vi "Real Time.vi"() -> ()   [LabVIEW 2022 SP3]
uses:
  ScanningControl/Motion Controllers/-MotionRoutines/MotionGlobals.vi
  <instrlib>/niScope/Controls/niScope input clock source.ctl
  ScanningControl/Pulsers/pulser.ctl
  ScanningControl/-ScanSystem/Controls/location.ctl
  ScanningControl/Motion Controllers/NI_controller/-NI_MotionRoutines/MotionSys.ctl
  <vilib>/Motion/FlexMotion/FunctionsVIs/Trajectory.llb/Load Acceleration/Deceleration.flx
  ScanningControl/-ScanSystem/Controls/ScanType2.ctl
  <vilib>/Utility/miscctls.llb/LVRectTypeDef.ctl
  <vilib>/ptbypt/NI_PtbyPt.lvlib
  <vilib>/picture/picture.llb/imagedata.ctl
  Annular Array/-AnnularRoutines/ArrayGeometry.ctl
  ScanningControl/Digitizers/-DigitizerRoutines/Digitizer.ctl
  <vilib>/Utility/miscctls.llb/LVBoundsTypeDef.ctl
  ScanningControl/Digitizers/-DigitizerRoutines/DigitizerGlobals.vi
  ScanningControl/Pulsers/PulserGlobals.vi
  Patient Routines/PatientGlobals.vi
  Annular Array/-AnnularRoutines/TransGeometry.ctl
  ScanningControl/Motion Controllers/Galil/Command Menu.ctl
  Annular Array/-AnnularRoutines/AnnularArray.ctl
panel:
  in  "Ann Array Params":T1={"Synth Foc?"=FALSE, "Focal Zones"=41, "Switch T/R"=0, "Trans Geometry (mm)"={"Transducer"=0, "Geo Focus"=12.0, "a (radius)"=3.0, "# of rings"=5, "kerf space "=0.1, "Center Freq"=12.0}, "Sub Ap Excite?"=FALSE, "Full Array Scan?"=FALSE, "Xmt/Rcv"={"XMIT"=[TRUE, TRUE, TRUE, TRUE, TRUE], "RCV"=[TRUE, TRUE, TRUE, TRUE, TRUE]}, "PulseSpacing (us)"=0.0, "Xmit Ring"=0, "XMIT CHS"=0, "RCV CHS"=0, "GPU?"=FALSE, "Save TIFF?"=FALSE, "downfactor"=1, "RCV 1CH"=0} {"RCV 1CH" items=["All", "1", "2", "3", "4", "5"]; "Trans Geometry (mm)"."Transducer" items=["6D 12R 40 MHz"=0, "10D 31R 20 MHz"=1, "10D 23R 20 MHz"=2, "6D 23R 40 MHz"=3, "4.5D 10.7R 40 MHz"=4, "9D 23.5R 20 MHz"=5, "9D 25.8R 20MHz"=6, "Enter"=99]; "Switch T/R" min=1 max=5 step=1}
  out "File Name":string="2015_000"
  in  "ExitSendCmd":bool
  in  "Sector":bool
  in  "Visible":bool
  in  "Center":bool
  in  "c (m/s)":dbl=1485.0
  out "append letter":i8=65
  in  "Scale (dB)":cluster{i32, i32}(slide)={-55, 0}
  out "Raw data":dbl[][](graph)
  in  "Tab Control":enum32{"Main Control", "Special Settings"}(tab)
  in  "Mode":T4(ring)
  in  "Save All Queue":bool
  out "fps":dbl format="%.1g"
  out "InQueue":i32
  in  "Patient Info":bool
  in  "Plane":i8(knob)=1 min=1 max=12 step=1 scale=0.0..12.0
  in  "View Queue":bool
  in  "Save All Real Time":bool
  in  "Save Raw":bool
  out "No data\nEntering\nQueue":bool
  in  "Pause":bool=TRUE
  in  "Flush Queue":bool
  in  "Image Scaling":T5(radio)
  in  "go":bool
  in  "Scan Location":enum32{"Radio Selection 1", "Radio Selection 2"}(radio)
  in  "Daxsonics Settings":T6={"Freq (MHz) "=20, "Amp (V)"=0, "Gain (dB)"=22} {"Freq (MHz)" items=["50"=50, "45"=45, "40"=40, "35"=35, "30"=30, "25"=25, "20"=20, "17"=17, "15"=15, "12"=12, "10"=10, "8"=8, "6"=6, "4"=4]; "Amp (V)" items=["100"=100, "95"=95, "90"=90, "85"=85, "80"=80, "75"=75, "70"=70, "65"=65, "60"=60, "55"=55, "50"=50, "45"=45, "40"=40, "35"=35, "30"=30, "25"=25, "20"=20, "15"=15, "10"=10, "0"=0]; "Gain (dB)" items=["45"=45, "42"=42, "39"=39, "36"=36, "33"=33, "30"=30, "27"=27, "24"=24, "21"=21, "18"=18, "15"=15, "12"=12, "9"=9, "6"=6, "3"=3, "0"=0]}
  out "Process backlog":i32
  in  "Accel":dbl(slide)=100.0 scale=1000000.0..7000000.0 scale format="%#_6e"
  in  "Adjust fps (%)":i16(slide)=100 min=0 max=150 step=5 scale=0.0..150.0
  in  "Xtra delay (us)":dbl=10.0
  in  "LowTime":dbl=0.01
  in  "Gate Length":dbl=0.19 format="%.6f"
  in  "Filter?":bool=TRUE
  in  "Dig Scale":dbl(ring)=0.4 items=["10 V"=10.0, "4 V"=4.0, "2 V"=2.0, "1 V"=1.0, "400 mV"=0.4, "200 mV"=0.2, "100 mV"=0.1]
  in  "RF data Sampling":T7={"Sampling Rate"=100.0, "Ref Delay (ms)"=0.0, "rf points per line"=2048} {"rf points per line" min=1; "Ref Delay (ms)" format="%.2f"}
  out "Frame":i32
  out "Sat Ct":u16(slide) scale=0.0..400.0
  in  "N":u8=100 min=1 max=100 step=1
  in  "Xmt/Rcv":cluster{"XMIT":bool[], "RCV":bool[]}={"XMIT"=[TRUE, TRUE, TRUE, TRUE, TRUE], "RCV"=[TRUE, TRUE, TRUE, TRUE, TRUE]}
  in  "Focal Zones":i16
  in  "GPU?":bool
  # "Ruler"
  # "© 2011-2015 Riverside Research Institute"
  # "Daxsonics"
  # "View"
  # "Data Archiving"
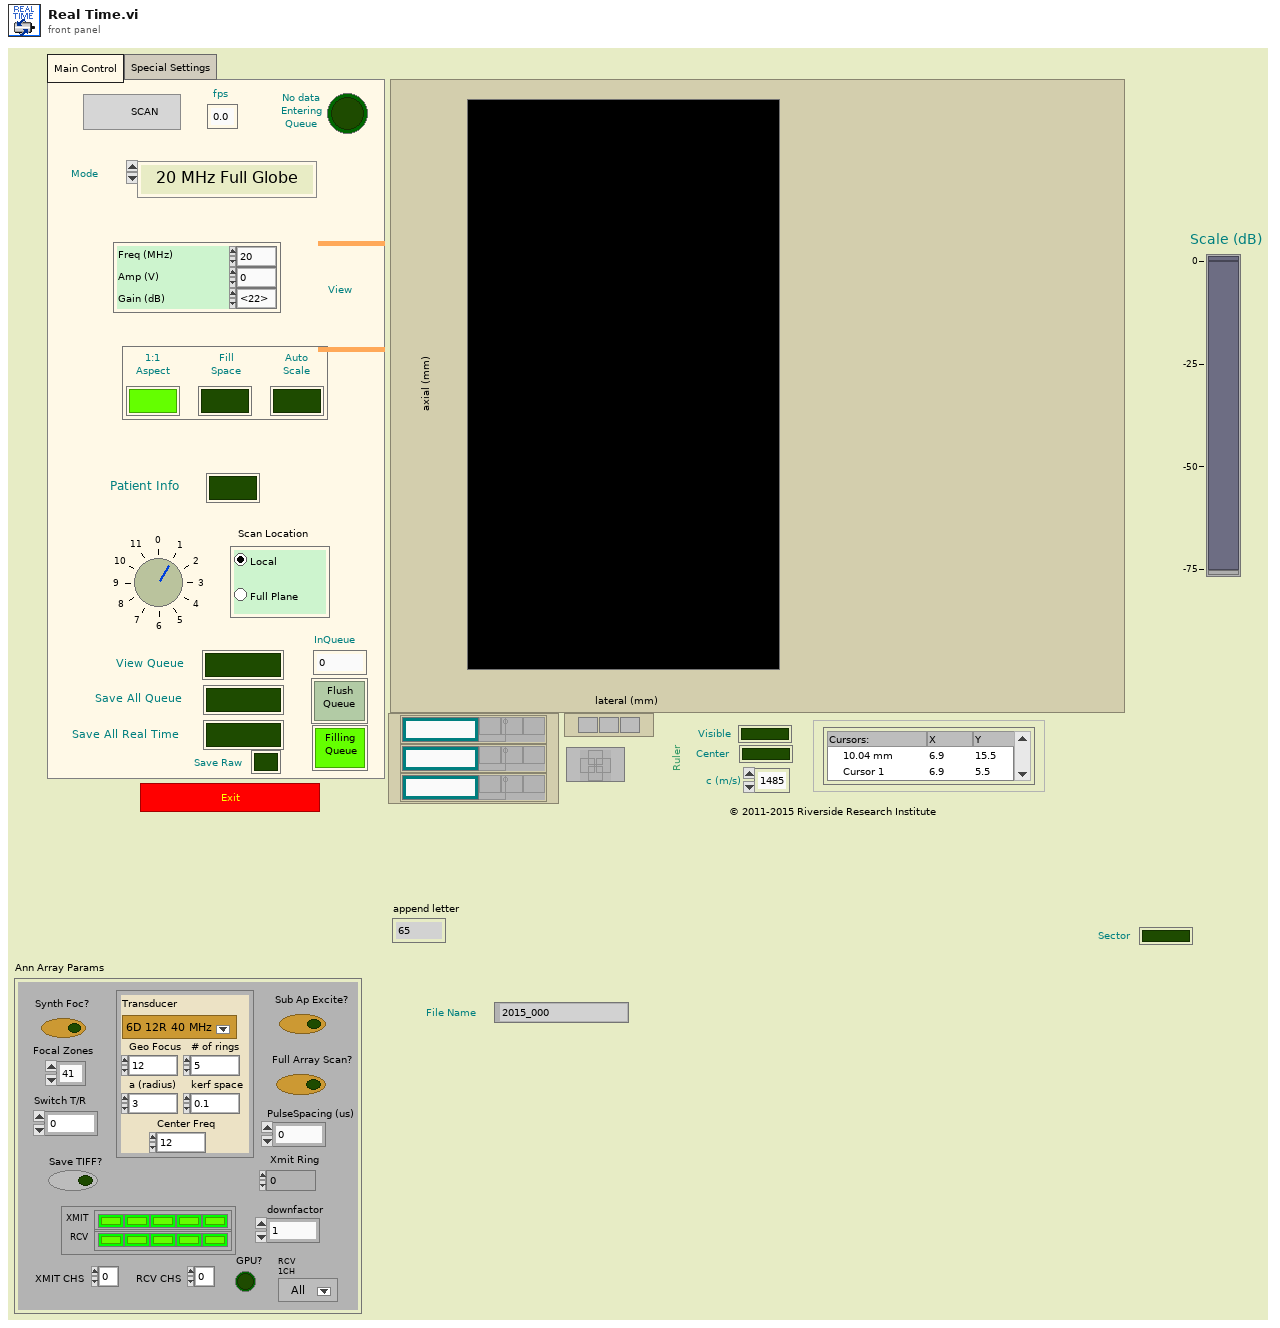
[diagram p1: front panel]
types:
  T1 = typedef "AnnularArray.ctl" = cluster{"Synth Foc?":bool, "Focal Zones":i16, "Switch T/R":i16, "Trans Geometry (mm)":T2, "Sub Ap Excite?":bool, "Full Array Scan?":bool, "Xmt/Rcv":cluster{"XMIT":bool[], "RCV":bool[]}, "PulseSpacing (us)":sgl, "Xmit Ring":i32, "XMIT CHS":u8, "RCV CHS":u8, "GPU?":bool, "Save TIFF?":bool, "downfactor":i32, "RCV 1CH":u16}
  T2 = typedef "TransGeometry.ctl" = cluster{"Transducer":T3, "Geo Focus":dbl, "a (radius)":dbl, "# of rings":i32, "kerf space ":dbl, "Center Freq":dbl}
  T3 = typedef "ArrayGeometry.ctl" = u16
  T4 = enum16{"20 MHz Full Globe", "20 MHz Anterior", "20 MHz Posterior", "New 20 MHz Full Globe", "New 20 MHz Anterior", "New 20 MHz Posterior", "F2 40 MHz", "F2 40 MHz Deep", "F3 20 MHz", "F3 20 MHz Deep", "Aviso Probe"}
  T5 = enum32{"1:1\nAspect", "Fill\nSpace", "Auto\nScale"}
  T6 = cluster{"Freq (MHz) ":u16, "Amp (V)":u16, "Gain (dB)":u16}
  T7 = cluster{"Sampling Rate":dbl, "Ref Delay (ms)":dbl, "rf points per line":i32}
  T8 = typedef "Digitizer.ctl" = enum16{"Acqiris Digitizer", "NI Digitizer", "LeCroy", "GaGe", "AlazarTech", "No Digitizer", "Teledyne"}
  T9 = typedef "LVBoundsTypeDef.ctl" = cluster{"Width":u32, "Height":u32}
  T10 = typedef "LVRectTypeDef.ctl" = cluster{"Left":i16, "Top":i16, "Right":i16, "Bottom":i16}
  T11 = typedef "pulser.ctl" = enum16{"Pan 5900", "Daxsonics", "Agilent 33xxx", "UTEX", "JSR", "WMC Mono-Cycle", "No Pulser", "NYU AVTECH", "Tabor W1281A", "Pan 5800", "Unlisted", "Tabor WX2182B"}
  T12 = typedef "MotionSys.ctl" = enum16{"MM3000", "NI 735x", "Newport ESP", "No Motion Card", "Galil"}
  T13 = typedef "location.ctl" = enum16{"Automatic", "WCM Main", "Hawaii", "Columbia MM3000", "Columbia  NI System", "NYU", "RRI 2", "UHI Allen", "CUMC RT", "Chiba", "Stony Brook", "WCM Microscopy", "WCM Aeoretch", "WCM Optics Lab", "WCM Main 2Axis", "WCM Rotation", "WCM SAM SMAC", "SERI GP"}
  T14 = typedef "DigitizerSettings.ctl" = cluster{"Digitizer delay (us) ":dbl, "rf points per line":i32, "lines per plane":i32, "Samp Rate (Hz)":dbl, "Additional dig delay (us)":dbl, "Voltage Scale":dbl, "Pre-Looks":i32, "Offset delay (us)":dbl, "bits A/D":i8, "Avg Num":i32, "DigTimeOut":sgl, "Rel Dig Delay":sgl, "Dig Ch":i32, "LeCroyCluster":cluster{"LeCroy Channels":bool[], "LC read pt offset":dbl, "Sweep Avg":bool}, "Main Digitizer":T8, "Dig Config":T15, "Digitizer ID Cluster":T16, "Trigger Settings":cluster{"Trig Source":u16, "Trig Coupling":u16, "Trig Slope":u16, "Level (mV)":dbl}, "Bulk Acq":bool, "Bulk Start Indexes":i32[], "Data Ref RF":refnum<data-value>, "NI ID/Channel":cluster{"NI ID":refnum<k15>, "NI CH":i32}[], "Total Dig CH":i32, "Xtra Ann Trig delay (us)":dbl, "Fix Z Delay?":bool, "One Way Transmission?":bool, "Data Ref Log":refnum<data-value>}
  T15 = typedef "DigConfig.ctl" = enum16{"Single channel", "2 Chans w/ 2 Acqiris", "2 Chans w/ 1 Acqiris", "5-CH Pulser New", "5-CH pulser w/ ann array", "5-pass style ann array", "Empty"}
  T16 = typedef "DigitizerID.ctl" = cluster{"Acqiris/Alazar/SP ID":u32[], "NI Instr Handles":refnum<k15>[], "LeCroy VISA":refnum<visa-resource-name>, "GaGe Handle":cluster{"Handle":u32, "Sample size":u32, "Resolution":i32, "Offset":i32, "Channels":u32, "Boards":u32}, "ATS Ref":string, "Acqiris Address":string[], "ADQRef":refnum<k24>, "adq_cu_ptr":refnum<k24>}
  T17 = cluster{"DataBufferQ":refnum<queue>, "LastNQ":refnum<queue>, "LastNBMPQ":refnum<queue>, "SaveRawN":refnum<notifier>, "StopN":refnum<notifier>}
  T18 = typedef "imagedata.ctl" = cluster{"image type":i32, "image depth":i32, "image":u8[], "mask":u8[], "colors":u32[], "Rectangle":cluster{"left":i16, "top":i16, "right":i16, "bottom":i16}}
  T19 = cluster{"gain":dbl, bool, "wfm":i16[][], "Sat Pts":i32, bool}
  T20 = cluster{"Source":u16, "Coupling":u16, "Slope":u16, "Level":dbl}
  T21 = typedef "ScanType2.ctl" = enum16{"Therapy With Scan", "M scan", "M Scan With Therapy Burst", "1-D B Scan", "1-D B Scan With Therapy Burst", "2-D B Scan", "2-D B Scan With Therapy Burst", "Rotational Scan", "1-D B-Scan PRF", "2-D B-Scan PRF", "Real-Time Scan", "Contrast Agents", "1-D w/ Real-Time Set Up", "Dual Transducer", "Acoustic Microscopy", "Hydrophone Scanning"}
  T22 = enum16{"Home", "Index", "Center", "Forward Limit", "Reverse Limit", "Run Sequence"}
  T23 = typedef "Command Menu.ctl" = enum16{"CommandPassThrough", "Abort Motion", "Define Pos", "Velocity", "Acceleration", "Deceleration", "Position Rel", "Postion Abs", "Begin Move", "KI", "KD", "KP", "IL", "Config I/O", "Set Bit", "Clear Bit", "Motor Off", "Moto On", "Status", "Execute", "Halt Execute", "HX Status", "Tell Velocity", "Check Motion", "BreakPoint", "Tell Position", "Current Code Line", "Tell Switches", "OC Force On", "OC Off"}
  T24 = cluster{"low cutoff":i32, "order":i32, "high cutoff":i32}
  T25 = cluster{"Source":u16, "Coupling":u16, "Slope":u16, "Level (mV)":dbl}
  T26 = cluster{"Voltage Scale":dbl, "Offset":dbl, "Coupling":u16}
  T27 = typedef "niScope input clock source.ctl" = u16
  T28 = typedef "LVStringsAndValuesArrayTypeDef_DBL.ctl" = cluster{"String":string, "Value":dbl}[]
  T29 = typedef "LVStringsAndValuesArrayTypeDef_U16.ctl" = cluster{"String":string, "Value":u16}[]
  T30 = typedef "Dax_Control_Cluster.ctl" = cluster{"Freq (MHz) ":u16, "Voltage (V)":u16, "Gain (dB)":u16}
  T31 = typedef "MotionParameters.ctl" = cluster{"No Motion?":bool, "Motion System":T12, "Motion Bd ID":u8, "Motion Profile":string, "# Axis":i8, "Reverse Z axis?":bool, "SMAC Axis":u16, "scan pair":T32, "RT fps":sgl, "Steps per mm":i32[], "Motor Parameters":cluster{"velocity ct/s":dbl[], "accel ct/s^2":dbl[]}, "One Way Scan":bool, "Reverse One Way Scan":bool, "Global Position (mm)":dbl[], "Plane":i32, "Distance between\nscan lines (um)":sgl, "Distance between\nscan planes (um)":sgl, "number of scan planes":i32, "Total steps in line":i32, "Xtra plane\ndistance  (um)":i32, "Xtra planes ":i32, "Add Axis":bool, "overshoot cts":i32, "BKPT Shift":i32, "Scan Start Time (ms)":u32, "ESP VISA":refnum<visa-resource-name>, "3rd Axis":T33, "GL Ref Out":refnum<k7>, "Galil Address":string}
  T32 = typedef "ScanAxis.ctl" = enum16{"y-(x) scan", "x-(y) scan", "z-(x) scan", "z-(y) scan", "y-(z) scan", "x-(z) scan", "w-(x) scan", "w-(y) scan", "w-(z) scan", "x-(w) scan", "y-(w) scan", "z-(w) scan"}
  T33 = typedef "3rdAxis.ctl" = u16
  T34 = typedef "Bd Id Out" = u8
  T35 = typedef "Resource Out (Enum).flx" = u16
  T36 = typedef "AxisOrVectorSpaceControl To Control.flx" = u16
  T37 = typedef "GL Axis Control.ctl" = u16
  T38 = cluster{"FIR Windowed Coefficients":dbl[], "Filter Prams":cluster{"low cutoff":i32, "order":i32, "high cutoff":i32}}
  T39 = cluster{"gain":dbl, bool, "wfm":i16[][], "max queue size (-1, unlimited)":i32, bool}
  T40 = cluster{"Y Scale Offset":dbl, "Y Scale Multi":dbl, "X Scale Offset":dbl, "X Scale Multi":dbl, "Gate Distance":dbl}
  T41 = typedef "PatientInfoDef.ctl" = cluster{"Eye Selector":enum32{"Left", "Right"}, "Plane":i8, "First Name":string, "Last Name":string, "Notes":string, "Patient ID":string, "Scan Location":enum32{"Radio Selection 1", "Radio Selection 2"}}
  T42 = typedef "LVPointDoubleTypeDef.ctl" = cluster{"Cursor X":dbl, "Cursor Y":dbl}
  T43 = typedef "LVRangeTypeDef.ctl" = cluster{"Minimum":dbl, "Maximum":dbl, "Increment":dbl, "Minor Increment":dbl, "Start":dbl}
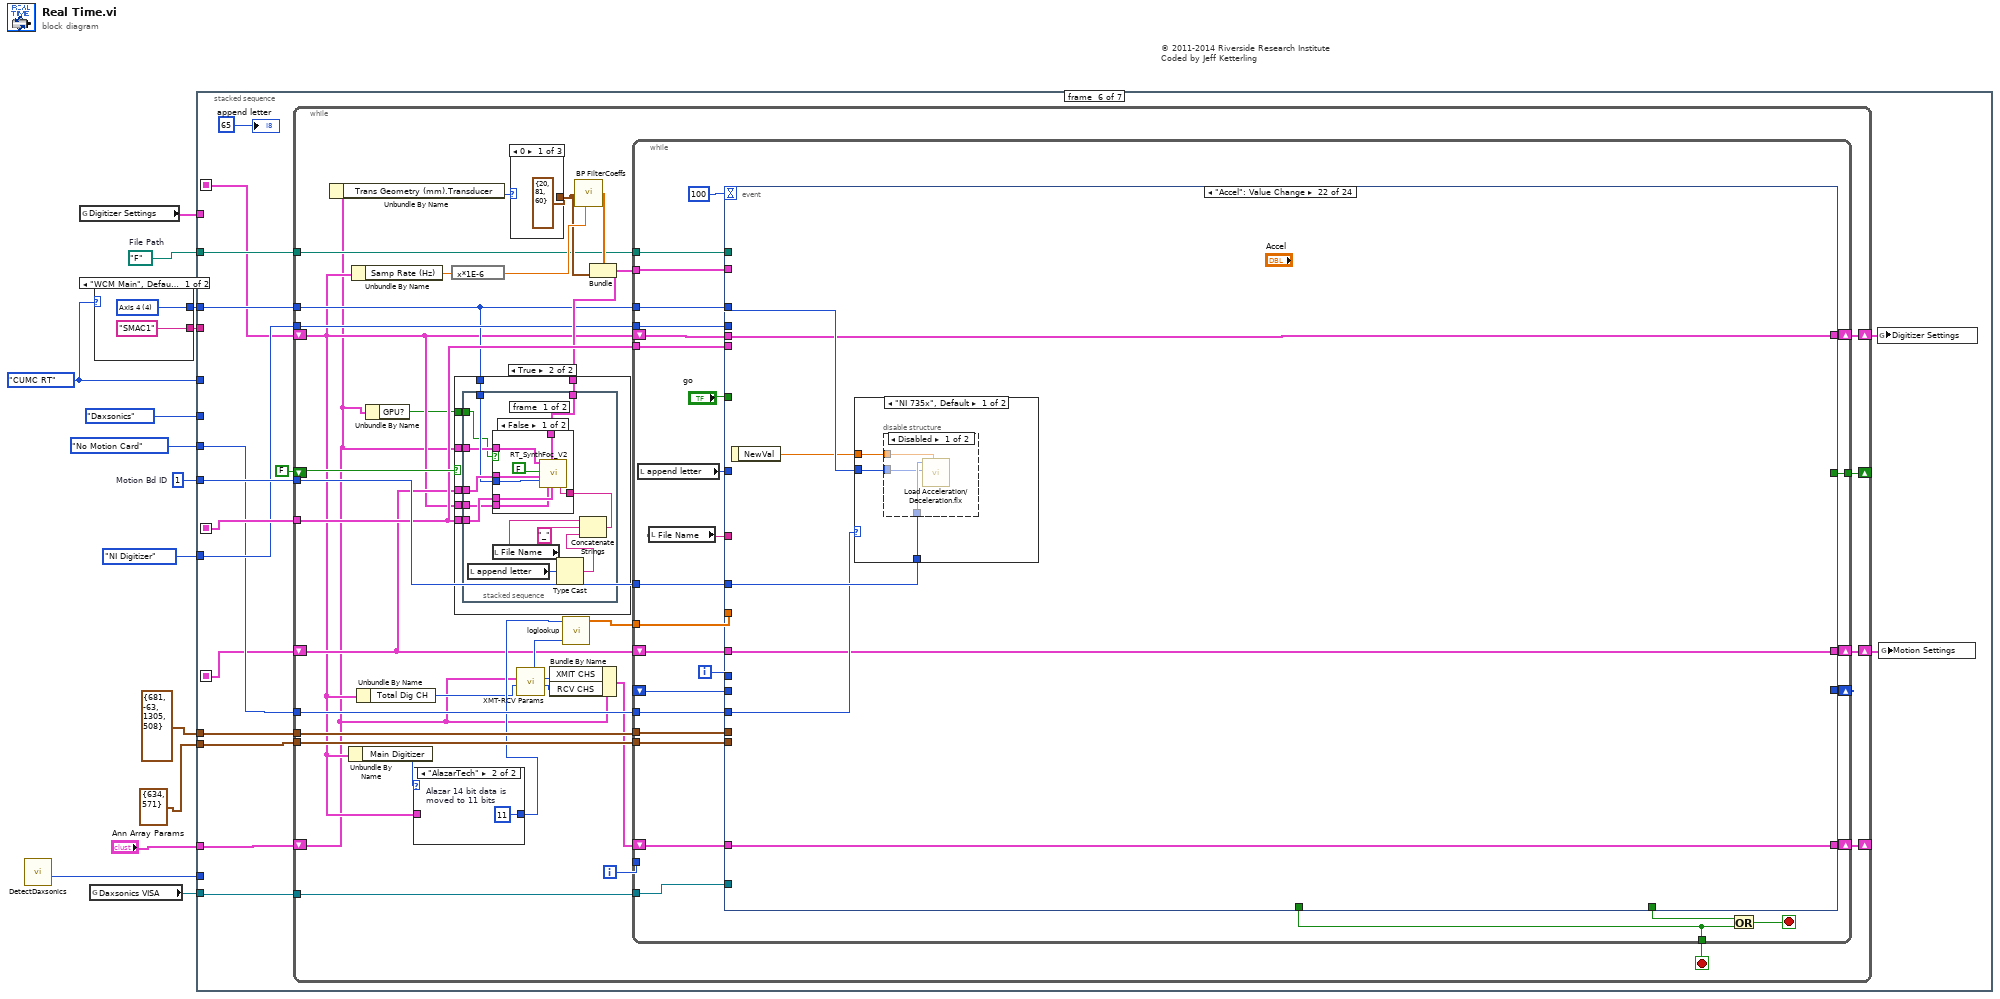
[diagram p0: block diagram]
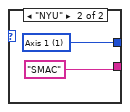
[diagram p2: hidden frame]
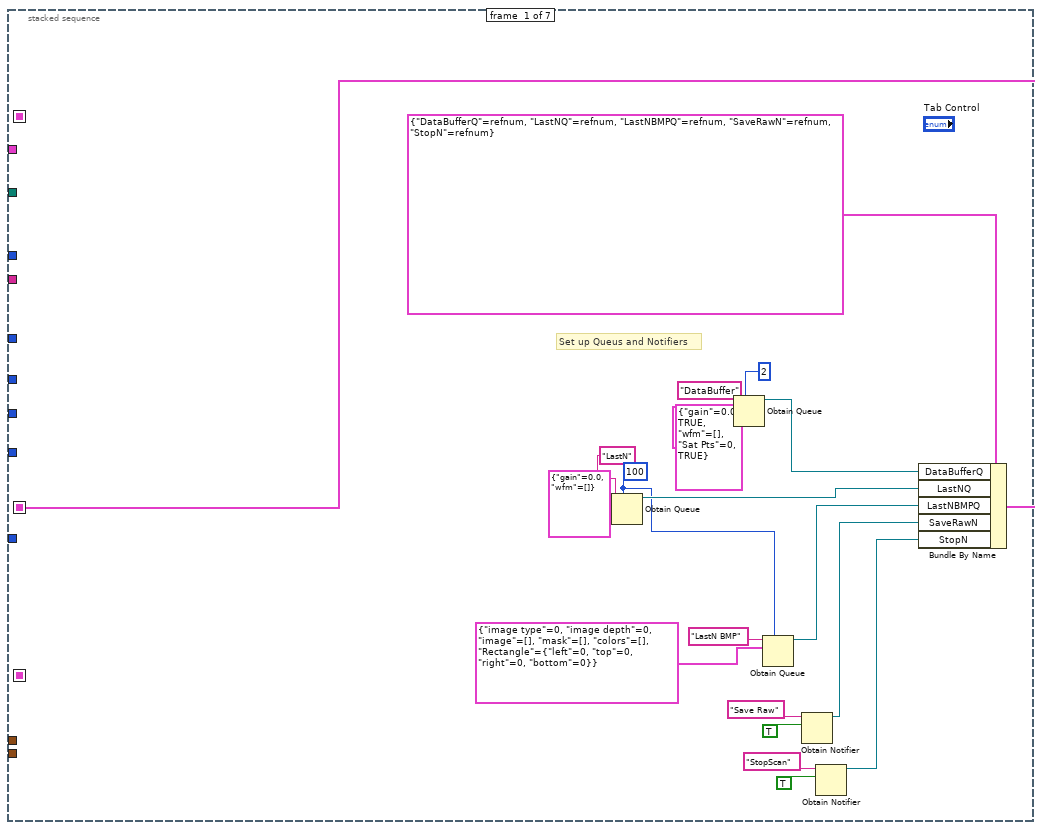
[diagram p3: hidden frame]
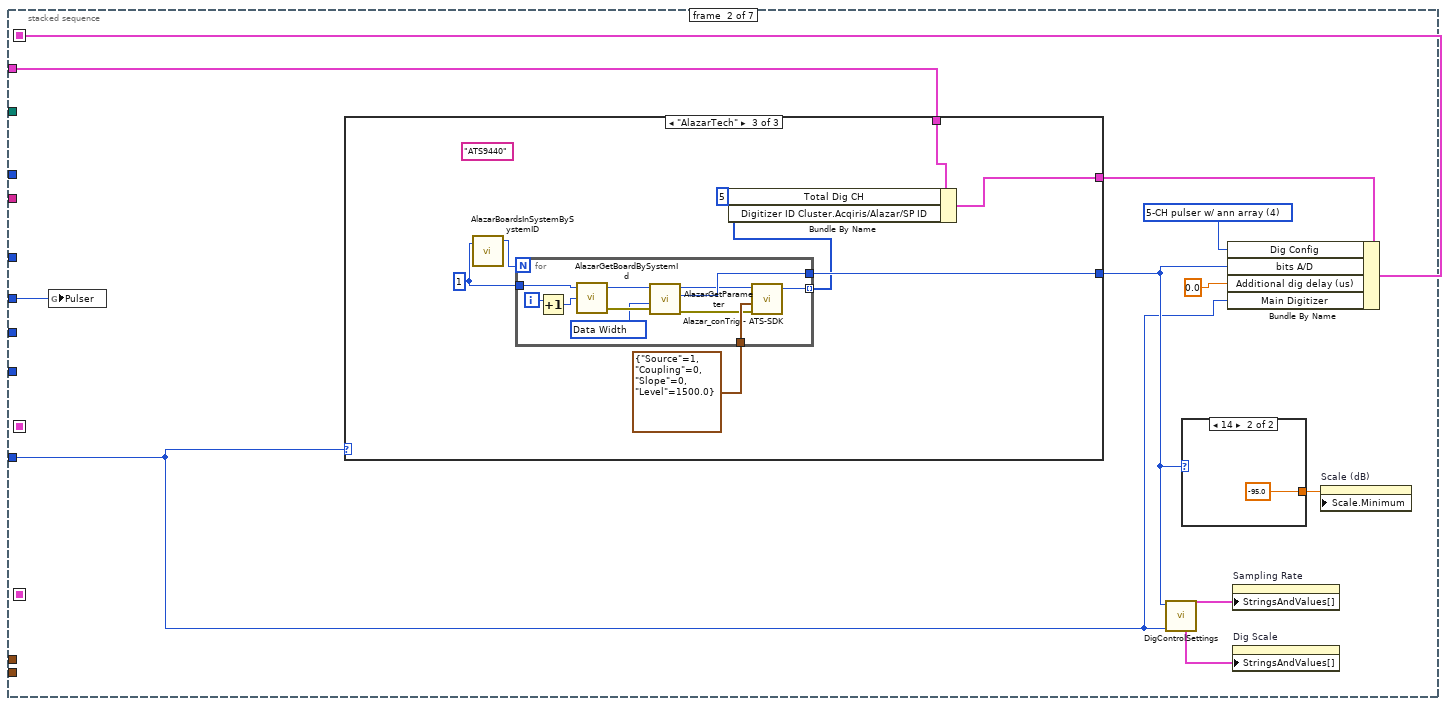
[diagram p4: hidden frame]
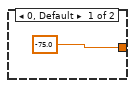
[diagram p5: hidden frame]
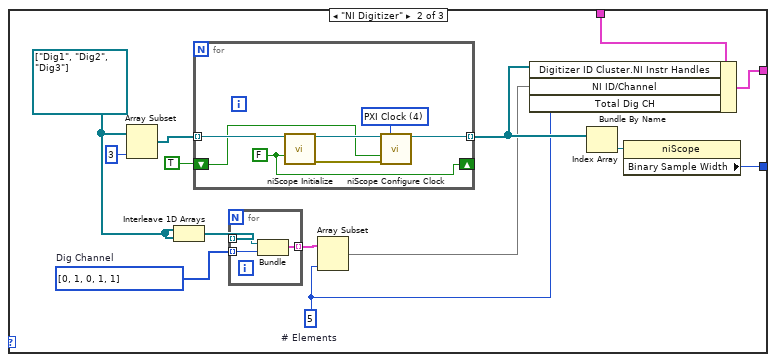
[diagram p7: hidden frame]
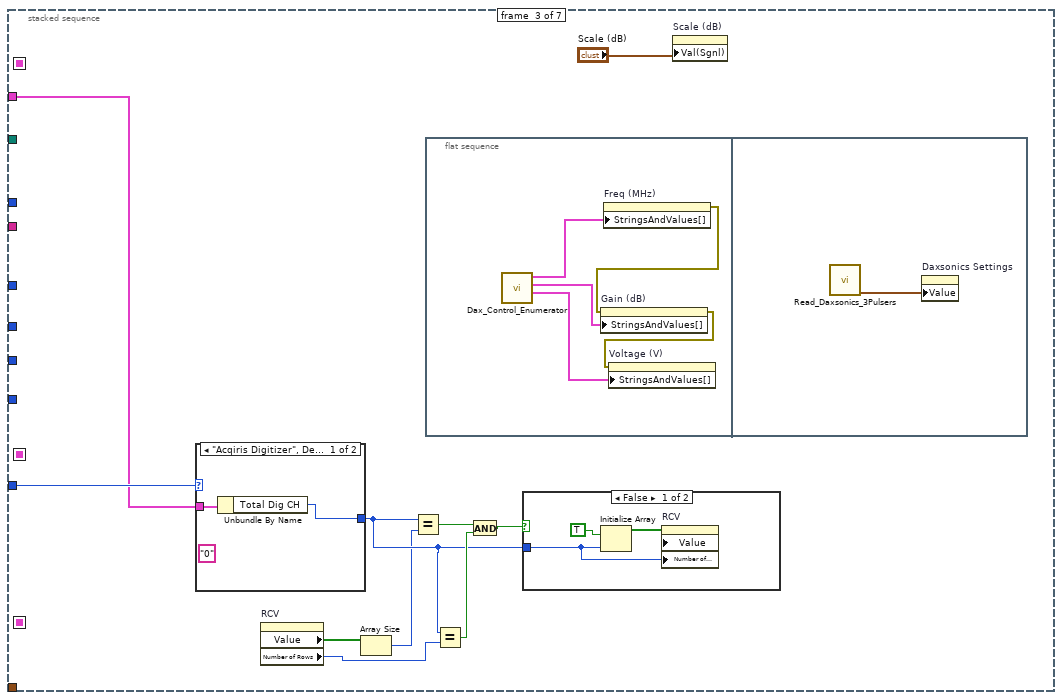
[diagram p8: hidden frame]
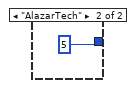
[diagram p10: hidden frame]
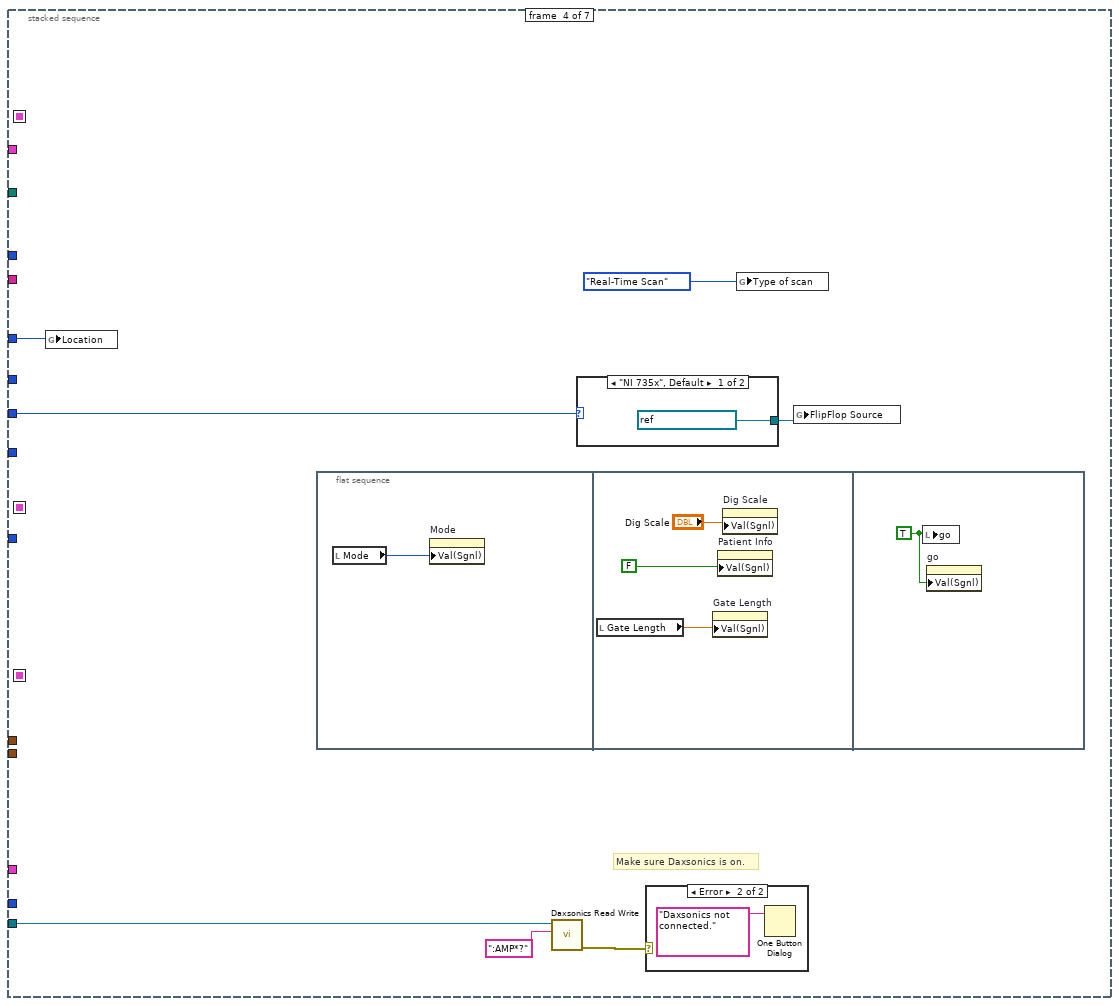
[diagram p11: hidden frame]
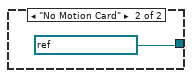
[diagram p12: hidden frame]
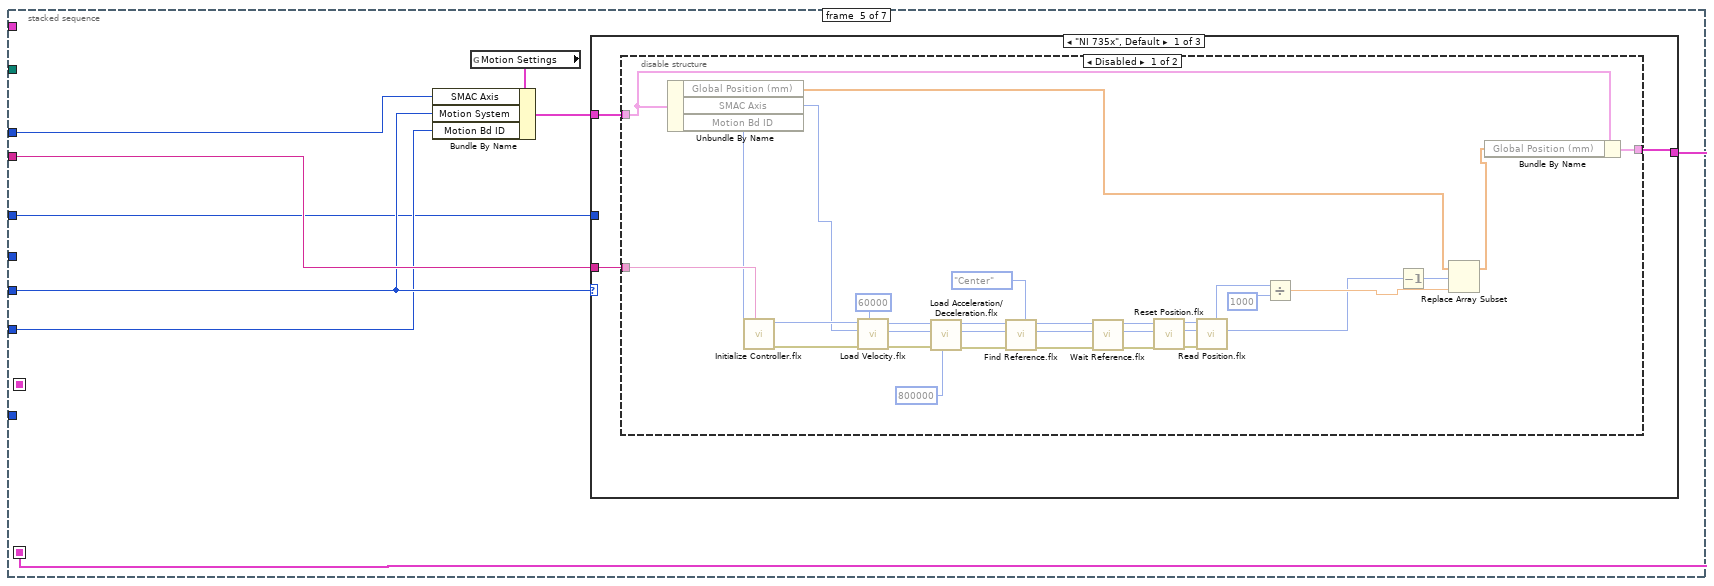
[diagram p14: hidden frame]
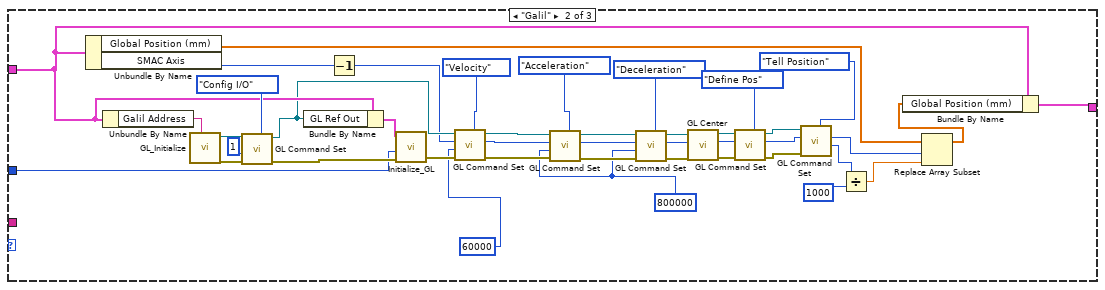
[diagram p16: hidden frame]
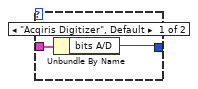
[diagram p18: hidden frame]
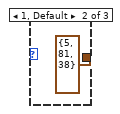
[diagram p19: hidden frame]
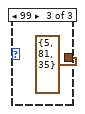
[diagram p20: hidden frame]
diagram:
  w8 = path "F:/"  # File Path
  w12 = location."CUMC RT" ("Location")
  w14 = u8 1  # Motion Bd ID
  # "© 2011-2014 Riverside Research Institute\nCoded by Jeff Ketterling"
  n1 = call "DetectDaxsonics.vi"() -> ("Trig Slope"=w2:u16)  [unwired: 10 in, 1 out]
  n2 = global read "DigitizerGlobals.vi" "Digitizer Settings"() -> (w7:T14)
  n3 = global read "PulserGlobals.vi" "Daxsonics VISA"() -> (w1:refnum<visa-resource-name>)
  n4 = case shown="\"WCM Main\", Default" w12 {
    tunnel: [w16 w18] -> w13
    tunnel: ["SMAC1" "SMAC"] -> w10
    frame "WCM Main", Default {
      w16 = u16 4 items=["Axis 1"=1, "Axis 2"=2, "Axis 3"=3, "Axis 4"=4, "Axis 5"=5, "Axis 6"=6, "Axis 7"=7, "Axis 8"=8, "Vector Space 1"=17, "Vector Space 2"=18, "Vector Space 3"=19, "Vector Space 4"=20] ("Axis")
    }
    frame "NYU" {
      w18 = u16 1 items=["Axis 1"=1, "Axis 2"=2, "Axis 3"=3, "Axis 4"=4, "Axis 5"=5, "Axis 6"=6, "Axis 7"=7, "Axis 8"=8, "Vector Space 1"=17, "Vector Space 2"=18, "Vector Space 3"=19, "Vector Space 4"=20] ("Axis")
    }
  }
  n5 = stacked-sequence {
    seq-local: [w24 _ _ _ _ _ _] -> [_ _ _ _ _ w226 w977]
    seq-local: [_ w44 _ _ _ _ _] -> [_ _ _ _ _ w222 w974]
    seq-local: [_ _ _ _ w133 _ _] -> [_ _ _ _ _ w221 _]
    tunnel: w14 -> [_ _ _ _ w135 w232 _]
    tunnel: MotionSys."No Motion Card" ("Motion System") -> [_ _ _ w117 w136 w224 _]
    tunnel: w12 -> [_ _ _ w121 w131 _ _]
    tunnel: T9 {"Width"=634, "Height"=571} ("Plot Area:Size") -> [_ _ _ _ _ w230 w985]
    tunnel: T10 {"Left"=681, "Top"=-63, "Right"=1305, "Bottom"=508} ("Plot Area Bounds") -> [_ _ _ _ _ w229 w986]
    tunnel: w13 -> [_ _ _ _ w137 w228 _]
    tunnel: Digitizer."NI Digitizer" ("Main Digitizer") -> [_ w40 w102 _ _ w225 w976]
    tunnel: w10 -> [_ _ _ _ w138 _ _]
    tunnel: w8 -> [_ _ _ _ _ w223 _]
    tunnel: w7 -> [_ w43 w94 _ _ _ _]
    tunnel: pulser."Daxsonics" ("Pulser") -> [_ w38 _ _ _ _ _]
    tunnel: "Ann Array Params" -> [_ _ _ _ _ w218 _]
    tunnel: w2 -> [_ _ _ _ _ _ _]
    tunnel: w1 -> [_ _ _ w116 _ w217 _]
    frame #0 {
      w19 = 100 ("max queue size (-1, unlimited)")
      # "Set up Queus and Notifiers"
      n6 = Obtain Queue ("LastN")(max queue size (-1, unlimited)=w19, name (unnamed)="LastN", element data type=cluster{"gain":dbl, "wfm":i16[][]} {"gain"=0.0, "wfm"=[]}) -> (queue out=w25:refnum<queue>)  [unwired: 2 in, 2 out]
      n7 = Obtain Queue(max queue size (-1, unlimited)=2, name (unnamed)="DataBuffer", element data type=T19 {"gain"=0.0, TRUE, "wfm"=[], "Sat Pts"=0, TRUE}) -> (queue out=w20:refnum<queue>)  [unwired: 2 in, 2 out]
      n8 = Obtain Queue ("LastNBMP")(max queue size (-1, unlimited)=w19, name (unnamed)="LastN BMP", element data type=T18 {"image type"=0, "image depth"=0, "image"=[], "mask"=[], "colors"=[], "Rectangle"={"left"=0, "top"=0, "right"=0, "bottom"=0}} ("Image Data")) -> (queue out=w23:refnum<queue>)  [unwired: 2 in, 2 out]
      n9 = Obtain Notifier ("Raw eye")(name (unnamed)="Save Raw", notification data type=TRUE) -> (notifier out=w26:refnum<notifier>)  [unwired: 2 in, 2 out]
      n10 = Obtain Notifier ("Stop Scan")(name (unnamed)="StopScan", notification data type=TRUE) -> (notifier out=w22:refnum<notifier>)  [unwired: 2 in, 2 out]
      n11 = Bundle By Name(cluster=T17 {"DataBufferQ"=refnum, "LastNQ"=refnum, "LastNBMPQ"=refnum, "SaveRawN"=refnum, "StopN"=refnum} ("Qs and Notis"), "DataBufferQ"=w20, "LastNQ"=w25, "LastNBMPQ"=w23, "SaveRawN"=w26, "StopN"=w22) -> (w24:T17)
    }
    frame #1 {
      w39 = 4 items=["Single channel"=0, "2 Chans w/ 2 Acqiris"=1, "2 Chans w/ 1 Acqiris"=2, "5-CH pulser w/ ann array"=4, "5-pass style ann array"=5] ("Dig Config")
      n12 = global write "PulserGlobals.vi" "Pulser"(w38) -> ()
      n13 = case shown="\"AlazarTech\"" w40 {
        tunnel: [_ w61 w79] -> w45
        tunnel: w43 -> [_ w58 w82]
        tunnel: [_ w59 w81] -> w42
        frame "Acqiris Digitizer", Default {
        }
        frame "NI Digitizer" {
          w51 = 5  # # Elements
          w57 = i32[] [0, 1, 0, 1, 1]  # Dig Channel
          w53 = refnum<k15>[] ["Dig1", "Dig2", "Dig3"]
          n14 = Array Subset(array=w53, length=3) -> (w63:refnum<k15>[])  [unwired: 1 in]
          n15 = Interleave 1D Arrays(w53, w53) -> (w55:refnum<k15>[])
          n16 = for {
            tunnel: [w71] -> w60 mode=indexing
            tunnel: w63 -> [w70] mode=indexing
            shift-right: [w68] -> _
            shift-left: TRUE ("master enabled") -> [w69]
            w68 = FALSE ("reset device")
            w74 = T27 4 items=["None"=0, "RTSI Clock"=1, "PFI 0"=6, "PFI 1"=2, "PFI 2"=3, "PXI Clock"=4, "External"=5, "Clock In"=7] ("input clock source")
            n17 = call <instrlib>:"niScope Initialize.vi"("resource name"=w70, "reset device"=w68) -> ("instrument handle"=w72:refnum<k15>, "error out"=w73:errorcluster)  [unwired: 2 in, 10 out]
            n18 = call <instrlib>:"niScope Configure Clock.vi"("instrument handle"=w72, "input clock source"=w74, "master enabled"=w69, "error in"=w73) -> ("instrument handle out"=w71:refnum<k15>)  [unwired: 2 in, 9 out]
          }
          n19 = for {
            tunnel: w55 -> [w67] mode=indexing
            tunnel: w57 -> [w66] mode=indexing
            tunnel: [w65] -> w56 mode=indexing
            n20 = Bundle("resource name"=w67, w66) -> (w65:cluster{"resource name":refnum<k15>, i32})  [unwired: 1 in]
          }
          n21 = Array Subset(array=w56, length=w51) -> (w52:cluster{"resource name":refnum<k15>, i32}[])  [unwired: 1 in]
          n22 = Bundle By Name(cluster=w58, "Digitizer ID Cluster.NI Instr Handles"=w60, "NI ID/Channel"=w52, "Total Dig CH"=w51) -> (w59:T14)
          n23 = Index Array(array=w60) -> (element=w64:refnum<k15>)  [unwired: 1 in]
          n24 = property class="niScope"(reference=w64) -> ("Binary Sample Width"=w61:i32)  [unwired: 1 in, 2 out]
        }
        frame "AlazarTech" {
          w76 = u32 1 ("System ID")
          (unwired) "ATS9440" ("BoardToVerify")
          n25 = call "AlazarBoardsInSystemBySystemID.vi"("System ID"=w76) -> ("Board Count"=w77:u32)  [unwired: 1 in, 2 out]
          n26 = for {
            N: w77 -> [_]
            tunnel: [w90] -> w79
            tunnel: T20 {"Source"=1, "Coupling"=0, "Slope"=0, "Level"=1500.0} ("Trigger") -> [w88]
            tunnel: w76 -> [w84]
            tunnel: [w83] -> w75 mode=indexing
            i -> [w86]
            w91 = u32 268435465 items=["Data Width"=268435465, "Set/Get Async BuffSize"=268435513, "Set/Get Async Buffcount"=268435520, "Get Data Format"=268435522, "Get Samples Per Timestamp Clock"=268435524, "Get Records Captured"=268435525, "Get Async Buffers Pending"=268435536, "Get Async Buffers Pending Full"=268435537, "Get Async Buffers Pending Empty"=268435538, "ECC Mode"=268435528, "Get Aux Input Level"=268435529, "Get Channels Per Board"=268435568, "Pack Mode"=268435570, "Get FPGA Temperature"=268435584] ("Parameter")
            n27 = Increment(x=w86) -> (x+1=w85:i32)
            n28 = call "AlazarGetBoardBySystemId.vi"("Board ID"=w85, "System ID"=w84) -> ("error out"=w92:errorcluster, "Handle"=w93:u64)  [unwired: 1 in, 1 out]
            n29 = call "AlazarGetParameter.vi"("error in (no error)"=w92, "Parameter"=w91, "Handle"=w93) -> ("error out"=w87:errorcluster, "Value"=w90:i32, "Handle"=w89:u64)  [unwired: 1 in, 1 out]
            n30 = call "Alazar_conTrig - ATS-SDK.vi"("error in (no error)"=w87, "Trigger"=w88, "Handle in"=w89) -> ("Handle_Out"=w83:u32)  [unwired: 2 in, 1 out]
          }
          n31 = Bundle By Name(cluster=w82, "Total Dig CH"=5, "Digitizer ID Cluster.Acqiris/Alazar/SP ID"=w75) -> (w81:T14)
        }
      }
      n32 = call "DigControlSettings.vi"(8:w40, 11:w45) -> ("Sampling Rates"=w47:T28, "Voltage Scale"=w48:T28)  [unwired: 5 in, 3 out]
      n33 = case shown="14" w45 {
        tunnel: [-75.0 ("Scale.Range:Maximum") -95.0 ("Scale.Range:Maximum")] -> w46
        frame 0, Default {
        }
        frame 14 {
        }
      }
      n34 = Bundle By Name(cluster=w42, "Dig Config"=w39, "bits A/D"=w45, "Additional dig delay (us)"=0.0 ("Additional dig delay (ms)"), "Main Digitizer"=w40) -> (w44:T14)
      n35 = property on="Sampling Rate" class="Ring (strict)"("StringsAndValues[]"=w47) -> ()  [unwired: 2 in, 2 out]
      n36 = property on="Dig Scale" class="Ring (strict)"("StringsAndValues[]"=w48) -> ()  [unwired: 2 in, 2 out]
      n37 = property on="Scale (dB)" class="Slide (strict)"("Scale.Minimum"=w46) -> ()  [unwired: 2 in, 2 out]
    }
    frame #2 {
      n38 = case shown="\"Acqiris Digitizer\", Default" w102 {
        tunnel: [w107 5] -> w98
        tunnel: w94 -> [w108 _]
        frame "Acqiris Digitizer", Default {
          (unwired) "0" ("Active Channel")
          n39 = Unbundle By Name(w108) -> ("Total Dig CH"=w107:i32)
        }
        frame "AlazarTech" {
        }
      }
      n40 = property on="RCV" class="Arr (strict)"() -> ("Value"=w103:bool[], "Number of Rows"=w96:u32)  [unwired: 2 in, 2 out]
      n41 = Array Size(array=w103) -> (size(s)=w97:i32)
      n42 = Equal?(x=w98, y=w97) -> (x = y?=w100:bool)
      n43 = flat-sequence {
        frame #0 {
          n44 = call "Dax_Control_Enumerator.vi"() -> ("Voltage"=w114:T29, "Gain"=w113:T29, "Freq"=w112:T29)  [unwired: 9 in]
          n45 = property on="Freq (MHz)" class="Ring (strict)"("StringsAndValues[]"=w112) -> (error out=w111:errorcluster)  [unwired: 2 in, 1 out]
          n46 = property on="Gain (dB)" class="Ring (strict)"(error in=w111, "StringsAndValues[]"=w113) -> (error out=w110:errorcluster)  [unwired: 1 in, 1 out]
          n47 = property on="Voltage (V)" class="Ring (strict)"(error in=w110, "StringsAndValues[]"=w114) -> ()  [unwired: 1 in, 2 out]
        }
        frame #1 {
          n48 = call "Read_Daxsonics_3Pulsers.vi"() -> ("Dax Values"=w115:T30)  [unwired: 5 in, 6 out]
          n49 = property on="Daxsonics Settings" class="Clust (strict)"("Value"=w115) -> ()  [unwired: 2 in, 2 out]
        }
      }
      n50 = Equal?(x=w98, y=w96) -> (x = y?=w101:bool)
      n51 = And(x=w100, y=w101) -> (x .and. y?=w99:bool)
      n52 = case shown="False" w99 {
        tunnel: w98 -> [w104 _]
        frame False {
          n53 = Initialize Array(TRUE, w104) -> (w105:bool[])
          n54 = property on="RCV" class="Arr (strict)"("Value"=w105, "Number of Columns"=w104) -> ()  [unwired: 2 in, 2 out]
        }
        frame True {
        }
      }
      n55 = property on="Scale (dB)" class="Slide (strict)"("Val(Sgnl)"="Scale (dB)") -> ()  [unwired: 2 in, 2 out]
    }
    frame #3 {
      # "Make sure Daxsonics is on."
      n56 = global write "MotionGlobals.vi" "Location"(w121) -> ()
      n57 = flat-sequence {
        frame #0 {
          n58 = local read "Mode"() -> (w123:T4)
          n59 = property on="Mode" class="Enum (strict)"("Val(Sgnl)"=w123) -> ()  [unwired: 2 in, 2 out]
        }
        frame #1 {
          n60 = local read "Gate Length"() -> (w126:dbl)
          n61 = property on="Gate Length" class="DigNum (strict)"("Val(Sgnl)"=w126) -> ()  [unwired: 2 in, 2 out]
          n62 = property on="Patient Info" class="Bool (strict)"("Val(Sgnl)"=FALSE ("Value (Signaling)")) -> ()  [unwired: 2 in, 2 out]
          n63 = property on="Dig Scale" class="Ring (strict)"("Val(Sgnl)"="Dig Scale") -> ()  [unwired: 2 in, 2 out]
        }
        frame #2 {
          w127 = TRUE ("go")
          n64 = local write "go"(w127) -> ()
          n65 = property on="go" class="Bool (strict)"("Val(Sgnl)"=w127) -> ()  [unwired: 2 in, 2 out]
        }
      }
      n66 = call "Daxsonics Read Write.vi"("write buffer"=":AMP*?", "VISA resource name"=w116) -> ("error out"=w120:errorcluster)  [unwired: 7 in, 2 out]
      n67 = case shown="\"NI 735x\", Default" w117 {
        tunnel: [refnum<k21> "Dev1 FlipFlop" ("FlipFlop Source") refnum<k21> "QuantFlipFlop" ("FlipFlop Source")] -> w118
        frame "NI 735x", Default {
        }
        frame "No Motion Card" {
        }
      }
      n68 = case shown="Error" w120 {
        frame No Error {
        }
        frame Error {
          n69 = One Button Dialog(message="Daxsonics not connected.") -> ()  [unwired: 1 in, 1 out]
        }
      }
      n70 = global write "MotionGlobals.vi" "Type of scan"(ScanType2."Real-Time Scan" ("Type of scan")) -> ()
      n71 = global write "MotionGlobals.vi" "FlipFlop Source"(w118) -> ()
    }
    frame #4 {
      n72 = global read "MotionGlobals.vi" "Motion Settings"() -> (w132:T31)
      n73 = Bundle By Name(cluster=w132, "SMAC Axis"=w137, "Motion System"=w136, "Motion Bd ID"=w135) -> (w134:T31)
      n74 = case shown="\"NI 735x\", Default" w136 {
        tunnel: w138 -> [w141 _ _]
        tunnel: w134 -> [w140 w203 w216]
        tunnel: [w139 w211 w216] -> w133
        tunnel: w131 -> [_ w174 _]
        frame "NI 735x", Default {
          n75 = disable-structure shown="Disabled" {
            disable-tunnel: w141 -> [w151 _]
            disable-tunnel: w140 -> [w145 _]
            disable-tunnel: [w142 _] -> w139
            frame Disabled {
              n76 = Unbundle By Name(w145) -> ("Global Position (mm)"=w144:dbl[], "SMAC Axis"=w147:u16, "Motion Bd ID"=w146:u8)
              n77 = call <vilib>:"Initialize Controller.flx"("Settings Name"=w151, "Board ID"=w146) -> ("error out"=w172:errorcluster, "Bd ID Out"=w173:T34)  [unwired: 1 in, 5 out]
              n78 = call <vilib>:"Load Velocity.flx"("Velocity (10000)"=60000 ("motor velocity"), "error in (no error)"=w172, "Axis or Vector Space"=w147, "Board ID"=w173) -> ("error out"=w169:errorcluster, "Resource Output"=w168:T35, "Bd ID Out"=w170:T34)  [unwired: 3 out]
              n79 = call "Load Acceleration/Deceleration.flx"("Acceleration (100000)"=800000 ("motor accel"), "error in (no error)"=w169, "Axis or Vector Space"=w168, "Board ID"=w170) -> ("error out"=w157:errorcluster, "Resource Output"=w153:T35, "Bd ID Out"=w158:T34)  [unwired: 1 in, 2 out]
              n80 = call <vilib>:"Find Reference.flx"("Search Type"=T22."Center", "error in (no error)"=w157, "Axis or Vector Space"=w153, "Board ID"=w158) -> ("error out"=w160:errorcluster, "Axis or Vector Space Output"=w159:T36, "Bd ID Out"=w161:T34)  [unwired: 5 in]
              n81 = call <vilib>:"Wait Reference.flx"("error in (no error)"=w160, "Axis or Vector Space"=w159, "Board ID"=w161) -> ("error out"=w155:errorcluster, "Axis or Vector Space Output"=w152:T36, "Bd ID Out"=w156:T34)  [unwired: 5 in, 1 out]
              n82 = call <vilib>:"Reset Position.flx"("error in (no error)"=w155, "Axis"=w152, "Board ID"=w156) -> ("error out"=w164:errorcluster, "Resource Output"=w166:T35, "Bd ID Out"=w165:T34)  [unwired: 4 in]
              n83 = call <vilib>:"Read Position.flx"("error in (no error)"=w164, "Axis"=w166, "Board ID"=w165) -> ("Resource Output"=w148:T35, "Position"=w163:i32)  [unwired: 5 out]
              n84 = Divide(x=w163, y=1000) -> (x/y=w149:dbl)
              n85 = Decrement(x=w148) -> (x-1=w150:T35)
              n86 = Replace Array Subset(array=w144, new element=w149, index=w150) -> (w143:dbl[])
              n87 = Bundle By Name(cluster=w145, "Global Position (mm)"=w143) -> (w142:T31)
            }
            frame Enabled {
            }
          }
        }
        frame "Galil" {
          w190 = 800000 ("motor accel")
          n88 = Unbundle By Name(w203) -> ("Global Position (mm)"=w213:dbl[], "SMAC Axis"=w192:u16)
          n89 = Unbundle By Name(w203) -> ("Galil Address"=w207:string)
          n90 = call "GL_Initialize.vi"("IP Address/COM"=w207) -> ("error out"=w205:errorcluster, "GL Ref Out"=w206:refnum<k7>)  [unwired: 5 in, 2 out]
          n91 = call "GL Command Set.vi"("Command"=Command_Menu."Config I/O", "error in (no error)"=w205, "Value"=1, "Galil.IGalil"=w206) -> ("error out"=w204:errorcluster, "ref out"=w193:refnum<k7>)  [unwired: 3 in, 3 out]
          n92 = Bundle By Name(cluster=w203, "GL Ref Out"=w193) -> (w210:T31)
          n93 = Decrement(x=w192) -> (x-1=w191:u16)
          n94 = call "Initialize_GL.vi"("Motion Settings"=w210, "Location"=w174, "error in"=w204) -> ("error out"=w194:errorcluster)  [unwired: 2 in, 2 out]
          n95 = call "GL Command Set.vi"("Command"=Command_Menu."Velocity", "error in (no error)"=w194, "Value"=60000 ("motor velocity"), "Axis"=w191, "Galil.IGalil"=w193) -> ("error out"=w201:errorcluster, "Axis Out"=w198:T37, "ref out"=w202:refnum<k7>)  [unwired: 2 in, 2 out]
          n96 = call "GL Command Set.vi"("Command"=Command_Menu."Acceleration", "error in (no error)"=w201, "Value"=w190, "Axis"=w198, "Galil.IGalil"=w202) -> ("error out"=w199:errorcluster, "Axis Out"=w197:T37, "ref out"=w200:refnum<k7>)  [unwired: 2 in, 2 out]
          n97 = call "GL Command Set.vi"("Command"=Command_Menu."Deceleration", "error in (no error)"=w199, "Value"=w190, "Axis"=w197, "Galil.IGalil"=w200) -> ("error out"=w187:errorcluster, "Axis Out"=w186:T37, "ref out"=w188:refnum<k7>)  [unwired: 2 in, 2 out]
          n98 = call "GL Center.vi"("error in"=w187, "Axis"=w186, "Galil.IGalil"=w188) -> ("error out"=w184:errorcluster, "Axis Out"=w182:T37, "Galil Out"=w185:refnum<k7>)  [unwired: 4 in]
          n99 = call "GL Command Set.vi"("Command"=Command_Menu."Define Pos", "error in (no error)"=w184, "Axis"=w182, "Galil.IGalil"=w185) -> ("error out"=w178:errorcluster, "Axis Out"=w180:T37, "ref out"=w179:refnum<k7>)  [unwired: 3 in, 2 out]
          n100 = call "GL Command Set.vi"("Command"=Command_Menu."Tell Position", "error in (no error)"=w178, "Axis"=w180, "Galil.IGalil"=w179) -> ("Response#"=w176:i32, "Axis Out"=w177:T37)  [unwired: 3 in, 3 out]
          n101 = Divide(x=w176, y=1000) -> (x/y=w214:dbl)
          n102 = Replace Array Subset(array=w213, new element=w214, index=w177) -> (w212:dbl[])
          n103 = Bundle By Name(cluster=w203, "Global Position (mm)"=w212) -> (w211:T31)
        }
        frame "No Motion Card" {
        }
      }
    }
    frame #5 {
      n104 = while {
        tunnel: w232 -> [w260]
        shift-right: [w265] -> _
        shift-left: FALSE ("go") -> [w266]
        tunnel: w230 -> [w262]
        tunnel: w229 -> [w261]
        tunnel: w228 -> [w241]
        tunnel: w217 -> [w258]
        tunnel: w226 -> [w256]
        tunnel: w225 -> [w251]
        tunnel: w224 -> [w249]
        tunnel: w223 -> [w248]
        shift-right: [w246] -> w219
        shift-left: w222 -> [w240]
        shift-right: [w242] -> w220
        shift-left: w221 -> [w243]
        shift-right: [w238] -> _
        shift-left: w218 -> [w233]
        i -> [w263]
        stop <- w264 stop-if-true
        n105 = Unbundle By Name(w233) -> ("Trans Geometry (mm).Transducer"=w250:T3)
        n106 = Unbundle By Name(w240) -> ("Main Digitizer"=w245:T8)
        n107 = Unbundle By Name(w240) -> ("Samp Rate (Hz)"=w247:dbl)
        n108 = Unbundle By Name(w240) -> ("Total Dig CH"=w239:i32)
        n109 = Unbundle By Name(w233) -> ("GPU?"=w234:bool)
        n110 = case shown="\"AlazarTech\"" w245 {
          tunnel: [w267 w269] -> w244
          tunnel: w240 -> [w268 _]
          frame "Acqiris Digitizer", Default {
            n111 = Unbundle By Name(w268) -> ("bits A/D"=w267:i8)
          }
          frame "AlazarTech" {
            w269 = 11  # Alazar 14 bit data is moved to 11 bits
          }
        }
        n112 = expression code="x*1E-6"(w247) -> (w257:dbl)
        n113 = case shown="0" w250 {
          tunnel: [T24 {"low cutoff"=20, "order"=81, "high cutoff"=60} ("Filter Prams") T24 {"low cutoff"=5, "order"=81, "high cutoff"=38} ("Filter Prams") T24 {"low cutoff"=5, "order"=81, "high cutoff"=35} ("Filter Prams")] -> w255
          frame 0 {
          }
          frame 1, Default {
          }
          frame 99 {
          }
        }
        n114 = call "XMT-RCV Params.vi"("Dig Channels"=w239, "Ann Array Params"=w233) -> ("# RCV"=w236:i16, "# XMIT"=w235:i16, "virtual T/R count"=w252:i16)  [unwired: 4 in, 3 out]
        n115 = Bundle By Name(cluster=w233, "XMIT CHS"=w235, "RCV CHS"=w236) -> (w237:T1)
        n116 = call "loglookup.vi"("A/D bits"=w244, "virtual T/R Pairs"=w252) -> ("Log Lookup"=w259:sgl[])  [unwired: 1 in, 3 out]
        n117 = call "BP FilterCoeffs.vi"("sample rate MHz"=w257, "Filter Prams"=w255) -> ("FIR Windowed Coefficients"=w254:dbl[])  [unwired: 4 in]
        n118 = Bundle("FIR Windowed Coefficients"=w254, "Filter Prams"=w255) -> (w253:T38)  [unwired: 1 in]
        n119 = case shown="True" w266 {
          tunnel: w256 -> [_ w279]
          tunnel: w253 -> [_ w278]
          tunnel: w240 -> [_ w277]
          tunnel: w243 -> [_ w276]
          tunnel: w241 -> [_ w275]
          tunnel: w233 -> [_ w274]
          tunnel: w234 -> [_ w273]
          frame False {
          }
          frame True {
            n120 = stacked-sequence {
              tunnel: w279 -> [w291 w312]
              tunnel: w278 -> [w285 _]
              tunnel: w277 -> [w284 _]
              tunnel: w276 -> [w283 _]
              tunnel: w275 -> [w282 _]
              tunnel: w274 -> [w281 _]
              tunnel: w273 -> [w280 _]
              frame #0 {
                n121 = local read "append letter"() -> (w287:i8)
                n122 = local read "File Name"() -> (w290:string)
                n123 = Type Cast(x=w287) -> (*(type *) &x=w286:string)  [unwired: 1 in]
                n124 = Concatenate Strings(w290, "_" ("string"), w286) -> (w289:string)
                n125 = case shown="False" w280 {
                  tunnel: w291 -> [w298 w305]
                  tunnel: w289 -> [w297 w304]
                  tunnel: w285 -> [w296 _]
                  tunnel: w284 -> [w295 w303]
                  tunnel: w283 -> [w294 w302]
                  tunnel: w282 -> [w293 w301]
                  tunnel: w281 -> [w292 w300]
                  frame False {
                    n126 = call "RT_SynthFoc_V2.vi"("Ann Array Params"=w292, "Pause?"=FALSE, "Motion Settings"=w294, "Scan Axis"=w293, "Digitizer Settings"=w295, "Filter"=w296, "Qs and Notis"=w298, "Raw Name"=w297) -> ()  [unwired: 10 in, 2 out]
                  }
                  frame True {
                    n127 = call "RT_SynthFoc_V2_GPU.vi"("Ann Array Params"=w300, "Pause?"=FALSE, "Motion Settings"=w302, "Scan Axis"=w301, "Digitizer Settings"=w303, "Qs and Notis"=w305, "Raw Name"=w304) -> ()  [unwired: 11 in, 2 out]
                  }
                }
              }
              frame #1 {
                n128 = Unbundle(w312) -> ("DataBufferQ"=w311:refnum<queue>, "LastNQ"=w310:refnum<queue>, "LastNBMPQ"=w309:refnum<queue>)  [unwired: 2 out]
                n129 = Flush Queue(queue=w311) -> (error out=w308:errorcluster)  [unwired: 1 in, 2 out]
                n130 = Flush Queue(queue=w310, error in (no error)=w308) -> (error out=w307:errorcluster)  [unwired: 2 out]
                n131 = Flush Queue(queue=w309, error in (no error)=w307) -> ()  [unwired: 3 out]
              }
            }
          }
        }
        n132 = while {
          tunnel: [w339] -> w265
          tunnel: [w336] -> w264
          tunnel: w263 -> [_]
          shift-right: [w335] -> _
          shift-left: _ -> [w334]
          tunnel: w262 -> [w333]
          tunnel: w261 -> [w332]
          tunnel: w260 -> [w331]
          tunnel: w241 -> [w330]
          tunnel: w259 -> [w328]
          tunnel: w258 -> [w327]
          tunnel: w256 -> [w326]
          tunnel: w253 -> [w324]
          tunnel: w251 -> [w323]
          tunnel: w249 -> [w322]
          tunnel: w248 -> [w321]
          shift-right: [w318] -> w246
          shift-left: w240 -> [w319]
          shift-right: [w316] -> w242
          shift-left: w243 -> [w317]
          shift-right: [w313] -> w238
          shift-left: w237 -> [w314]
          i -> [w315]
          stop <- w337 stop-if-true
          n133 = local read "append letter"() -> (w329:i8)
          n134 = local read "File Name"() -> (w320:string)
          n135 = event shown="[21] \"Accel\": Value Change" {
            selector: _ -> [_ _ _ _ _ _ _ _ _ _ _ _ _ _ _ _ _ _ _ _ _ _ _ _]
            dyn-events: _ -> [_ _ _ _ _ _ _ _ _ _ _ _ _ _ _ _ _ _ _ _ _ _ _ _]
            timeout: 100 -> [_ _ _ _ _ _ _ _ _ _ _ _ _ _ _ _ _ _ _ _ _ _ _ _]
            tunnel: w315 -> [w356 _ _ _ _ _ _ _ _ _ _ _ _ _ _ _ _ _ _ _ _ _ _ _]
            tunnel: w320 -> [w360 _ _ _ _ _ _ _ _ _ _ w810 w834 _ _ _ _ _ _ _ _ _ _ _]
            tunnel: [FALSE ("go") w441 _ w688 w709 _ w756 _ _ _ _ _ _ _ _ _ _ _ _ _ _ _ _ _] -> w339
            tunnel: [_ w441 _ w688 w709 _ w756 _ _ _ _ _ _ _ _ _ _ _ _ _ _ _ _ _] -> w338
            tunnel: [_ _ _ _ _ _ _ "ExitSendCmd" _ _ _ _ _ _ _ _ _ _ _ _ _ _ _ _] -> w336
            tunnel: [w358 _ _ _ _ _ _ _ _ _ _ _ _ _ _ _ _ _ _ _ _ _ _ _] -> w335
            tunnel: w334 -> [w357 _ _ _ _ _ _ _ _ _ _ _ _ _ _ _ _ _ _ _ _ _ _ _]
            tunnel: w333 -> [_ _ _ _ _ _ _ _ _ _ _ _ _ _ _ _ _ _ w894 _ _ _ _ _]
            tunnel: w332 -> [_ _ _ _ _ _ _ _ _ _ _ _ _ _ _ _ _ _ w893 _ _ _ _ _]
            tunnel: w331 -> [_ _ _ _ _ _ _ _ _ _ _ _ _ _ _ _ _ _ _ _ w942 w955 _ _]
            tunnel: w330 -> [_ _ _ w681 _ _ _ _ _ _ _ _ _ _ _ _ _ _ _ _ w941 w954 _ _]
            tunnel: w329 -> [w351 _ _ _ _ _ _ _ _ _ _ w813 w831 w839 _ _ _ _ _ _ _ _ _ _]
            tunnel: w328 -> [w353 _ _ _ _ _ _ _ _ _ _ _ _ _ _ _ _ _ _ _ _ _ _ _]
            tunnel: w327 -> [_ _ _ _ _ _ _ _ _ _ _ _ _ _ _ _ _ _ _ _ _ _ _ _]
            tunnel: w326 -> [w344 w440 _ w665 w713 _ w760 w773 _ _ _ w814 w832 _ w850 _ _ _ _ _ _ _ _ w973]
            tunnel: "go" -> [_ _ _ w688 w709 _ w757 _ _ _ _ _ _ _ _ _ _ _ _ _ _ _ _ _]
            tunnel: w324 -> [w350 _ _ _ _ _ _ _ _ _ _ _ _ _ _ _ _ _ _ _ _ _ _ _]
            tunnel: w323 -> [_ _ w476 _ w708 _ _ _ _ _ _ _ _ _ _ _ _ _ _ _ _ _ w965 _]
            tunnel: w322 -> [_ _ _ _ _ _ _ _ _ _ _ _ _ _ _ _ _ _ _ _ w940 w952 _ _]
            tunnel: w321 -> [_ _ _ _ _ _ _ _ _ w795 _ _ _ _ _ _ _ _ _ _ _ _ _ _]
            tunnel: w319 -> [w343 w438 w464 w686 w706 w750 w755 w771 w779 w792 w804 w809 w825 w837 w844 w855 w869 w875 w891 w931 w939 w951 w964 w970]
            tunnel: [w343 w438 w465 w667 w707 w750 w755 w771 w779 w792 w804 w809 w825 w837 w844 w855 w869 w875 w891 w931 w939 w951 w964 w970] -> w318
            tunnel: w317 -> [w342 w437 w462 w666 w705 w749 w754 w770 w780 w791 w803 w808 w824 w836 w843 w854 w868 w874 w890 w930 w938 w950 w963 w969]
            tunnel: [w342 w437 w459 w670 w705 w749 w754 w770 w780 w791 w803 w808 w824 w836 w843 w854 w868 w874 w890 w930 w938 w950 w963 w969] -> w316
            tunnel: w314 -> [w341 w436 w450 w664 w704 w747 w753 w769 w778 w790 w800 w807 w823 w835 w842 w853 w867 w873 w889 w929 w937 w949 w962 w968]
            tunnel: [w341 w436 w449 w664 w704 w747 w751 w769 w778 w790 w800 w807 w823 w835 w842 w853 w867 w873 w889 w929 w937 w949 w962 w968] -> w313
            event Timeout {
              n136 = event-data() -> ()  [unwired: 1 in, 1 out]
              n137 = Unbundle By Name(w344) -> ("DataBufferQ"=w352:refnum<queue>)
              n138 = Get Queue Status(queue=w352) -> (queue out=w355:refnum<queue>, # elements in queue=→"Process backlog":i32)  [unwired: 2 in, 6 out]
              n139 = Dequeue Element(queue=w355, timeout in ms (-1)=1000) -> (element=w349:T39, timed out?=w348:bool)  [unwired: 1 in, 2 out]
              n140 = Unbundle(w349) -> (w346:bool)  [unwired: 4 out]
              n141 = Or(x=w348, y=w346) -> (x .or. y?=w345:bool)
              "No data\nEntering\nQueue" <- w345
              n142 = case shown="False" w345 {
                tunnel: w356 -> [w379 _]
                tunnel: w360 -> [w388 _]
                tunnel: w349 -> [w400 _]
                tunnel: [w382 w435] -> w358
                tunnel: w357 -> [w378 w435]
                tunnel: w353 -> [w394 _]
                tunnel: w351 -> [w386 _]
                tunnel: w350 -> [w383 _]
                tunnel: w344 -> [w368 _]
                tunnel: w341 -> [w364 _]
                frame False {
                  # "20log(abs(x) of binary values up to 25*2^7"
                  # "Get and display data"
                  n143 = Unbundle By Name(w368) -> ("LastNQ"=w367:refnum<queue>, "LastNBMPQ"=w366:refnum<queue>)
                  n144 = Unbundle(w400) -> ("gain"=w395:dbl, w398:bool, "wfm"=w399:i16[][], "max queue size (-1, unlimited)"=→"Sat Ct":i32)  [unwired: 1 out]
                  n145 = Unbundle By Name(w364) -> ("GPU?"=w363:bool)
                  n146 = case shown="False" w398 {
                    tunnel: w399 -> [w432 w434]
                    tunnel: [w432 w433] -> w377
                    frame False {
                    }
                    frame True {
                      n147 = call "ReverseData.vi"("Array in"=w434) -> ("Array out"=w433:i16[][])
                    }
                  }
                  n148 = Type Cast(x=w386) -> (*(type *) &x=w385:string)  [unwired: 1 in]
                  n149 = Not(x=w363) -> (.not. x?=w365:bool)
                  n150 = invoke on="Raw data" class="IntGraph (strict)" method="Get Image"("image depth"=24) -> ("image data"=w391:T18)  [unwired: 5 in, 5 out]
                  n151 = And(x="Filter?", y=w365) -> (x .and. y?=w361:bool)
                  n152 = Get Queue Status(queue=w367) -> (queue out=w375:refnum<queue>, # elements in queue=→"InQueue":i32)  [unwired: 2 in, 6 out]
                  n153 = case shown="False" w361 {
                    tunnel: [w420 w423] -> w393
                    tunnel: w377 -> [w420 w422]
                    tunnel: w383 -> [_ w421]
                    frame False {
                    }
                    frame True {
                      n154 = call "BP FilterI16_Fast.vi"("Filter"=w421, "Array in"=w422) -> ("Filtered X"=w423:dbl[][])  [unwired: 4 in]
                    }
                  }
                  n155 = Bundle("gain"=w395, "Array out"=w377) -> (w396:cluster{"gain":dbl, "Array out":i16[][]})  [unwired: 1 in]
                  n156 = Concatenate Strings(w388, "_" ("string"), w385) -> (w390:string)
                  n157 = case shown="True" "Pause" {
                    tunnel: w375 -> [_ w404]
                    tunnel: w396 -> [_ w403]
                    tunnel: w366 -> [_ w402]
                    tunnel: w391 -> [_ w401]
                    frame False {
                    }
                    frame True {
                      n158 = Lossy Enqueue Element(queue=w404, element=w403) -> ()  [unwired: 1 in, 4 out]
                      n159 = Lossy Enqueue Element(queue=w402, element=w401) -> ()  [unwired: 1 in, 4 out]
                    }
                  }
                  n160 = case shown="False" "Sector" {
                    tunnel: w394 -> [w407 _]
                    tunnel: w393 -> [w406 w416]
                    tunnel: [w405 w415] -> w381
                    frame False {
                      n161 = for {
                        tunnel: [w410] -> w405 mode=indexing
                        tunnel: w407 -> [w409]
                        tunnel: w406 -> [w408] mode=indexing
                        n162 = for {
                          tunnel: [w414] -> w410 mode=indexing
                          tunnel: w409 -> [w413]
                          tunnel: w408 -> [w412] mode=indexing
                          n163 = Absolute Value(x=w412) -> (abs(x)=w411:dbl)
                          n164 = Index Array(array=w413, index=w411) -> (element=w414:sgl)
                        }
                      }
                    }
                    frame True {
                      n165 = call "AvisoSectorConvert.vi"("Raw In"=w416) -> ("Sector out"=w415:dbl[][])  [unwired: 10 in]
                    }
                  }
                  n166 = case shown="True" "Save All Real Time" {
                    tunnel: w377 -> [_ w431]
                    tunnel: 11 -> [_ w430]
                    tunnel: w379 -> [_ w429]
                    tunnel: w395 -> [_ w428]
                    tunnel: w390 -> [_ w427]
                    tunnel: w364 -> [_ w426]
                    frame False {
                    }
                    frame True {
                      n167 = call "RT_Save_EYE.vi"("Ann Array Params"=w426, "Digitizer Gain"=w428, "bits A/D"=w430, "Eye Name"=w427, "Frame"=w429, "Data"=w431) -> ()  [unwired: 6 in]
                    }
                  }
                  n168 = case shown="True" "Save All Real Time" {
                    tunnel: w391 -> [_ w419]
                    tunnel: w379 -> [_ w418]
                    tunnel: w390 -> [_ w417]
                    frame False {
                    }
                    frame True {
                      n169 = call "RT_Save_JPG.vi"("Movie Name"=w417, "Frame"=w418, "image data"=w419) -> ()  [unwired: 9 in]
                    }
                  }
                  n170 = Subtract(x=w382, y=w378) -> (x-y=w373:u32)
                  n171 = To Double Precision Float(number=w373) -> (double precision float=w372:dbl)
                  n172 = flat-sequence {
                    tunnel: w381 -> [w424]
                    tunnel: [w425] -> w382
                    frame #0 {
                      "Raw data" <- w424
                    }
                    frame #1 {
                      n173 = Tick Count (ms)() -> (millisecond timer value=w425:u32)
                    }
                  }
                  n174 = expression code="1000/x"(w372) -> (w371:dbl)
                  n175 = call <vilib>:"Mean PtByPt.vi"("x"=w371, "sample length"=10) -> ("mean"=→"fps":dbl)  [unwired: 2 in, 1 out]
                  "Frame" <- w379
                }
                frame True {
                }
              }
            }
            event "go": Value Change {
              n176 = event-data() -> ("NewVal"=w441:bool)  [unwired: 1 in, 4 out]
              n177 = Unbundle By Name(w440) -> ("StopN"=w439:refnum<notifier>)
              n178 = case shown="False" w441 {
                tunnel: w439 -> [w442 _]
                frame False {
                  n179 = flat-sequence {
                    tunnel: w442 -> [w443]
                    frame #0 {
                      n180 = Send Notification(notification=TRUE, notifier=w443) -> ()  [unwired: 1 in, 2 out]
                    }
                    frame #1 {
                      n181 = Wait (ms)(milliseconds to wait=u32 1000) -> ()  [unwired: 1 out]
                    }
                  }
                }
                frame True {
                }
              }
            }
            event "Mode", "Xtra delay (us)", "Focal Zones", "GPU?": Value Change {
              # "Scale Parameters"
              # "MotionGlobals.videlay mics"
              # "RF Points"
              # "Sampling"
              # "RF lines"
              n182 = event-data() -> ()  [unwired: 1 in, 6 out]
              n183 = case shown="\"F3 20 MHz\"" "Mode" {
                tunnel: [100000000.0 125000000.0 100000000.0 100000000.0 125000000.0 125000000.0 100000000.0 200000000.0 100000000.0 100000000.0 200000000.0] -> w468
                tunnel: [4000 2500 2400 4000 2500 2400 3000 4500 5000 6500 2000] -> w467
                tunnel: [139 139 139 139 139 139 281 281 211 211 101] -> w469
                tunnel: [18.666667 26.666667 34.666667 4.0 11.0 17.5 10.6667 10.6667 20.0 20.0 11.0] -> w466
                tunnel: [sgl 117.0 sgl 117.0 sgl 117.0 sgl 117.0 sgl 117.0 sgl 117.0 sgl 50.0 sgl 50.0 sgl 100.0 sgl 100.0 sgl 25.0] -> w457
                tunnel: [w499 w514 w529 w544 w559 w574 w591 w606 w621 w636 w649] -> w451
                tunnel: [sgl 10.0 sgl 10.0 sgl 10.0 sgl 10.0 sgl 10.0 sgl 10.0 sgl 10.0 sgl 10.0 sgl 10.0 sgl 10.0 sgl 8.0] -> w460
                tunnel: [200 200 200 200 200 200 200 200 200 200 200] -> w461
                tunnel: [5.0 ("Xtra delay (us)") 5.0 ("Xtra delay (us)") 5.0 ("Xtra delay (us)") 5.0 ("Xtra delay (us)") 5.0 ("Xtra delay (us)") 5.0 ("Xtra delay (us)") 10.0 ("Xtra delay (us)") 10.0 ("Xtra delay (us)") 15.0 ("Xtra delay (us)") 10.0 ("Xtra delay (us)") 0.0 ("Xtra delay (us)")] -> _
                tunnel: [bool[] [TRUE, TRUE, TRUE, TRUE, FALSE] ("RCV") bool[] [TRUE, TRUE, TRUE, TRUE, FALSE] ("RCV") bool[] [TRUE, TRUE, TRUE, TRUE, FALSE] ("RCV") bool[] [TRUE, TRUE, TRUE, TRUE, FALSE] ("RCV") bool[] [TRUE, TRUE, TRUE, TRUE, FALSE] ("RCV") bool[] [TRUE, TRUE, TRUE, TRUE, FALSE] ("RCV") bool[] [TRUE, TRUE, TRUE, TRUE, FALSE] ("RCV") bool[] [TRUE, TRUE, TRUE, TRUE, FALSE] ("RCV") bool[] [TRUE, TRUE, TRUE, TRUE, FALSE] ("RCV") bool[] [TRUE, TRUE, TRUE, TRUE, FALSE] ("RCV") bool[] [TRUE, TRUE, TRUE, TRUE, TRUE] ("XMIT")] -> w453
                tunnel: [bool[] [TRUE, TRUE, FALSE, FALSE, TRUE] ("XMIT") bool[] [TRUE, TRUE, TRUE, FALSE, TRUE] ("XMIT") bool[] [TRUE, TRUE, FALSE, FALSE, TRUE] ("XMIT") bool[] [TRUE, TRUE, FALSE, FALSE, TRUE] ("XMIT") bool[] [TRUE, TRUE, TRUE, FALSE, TRUE] ("XMIT") bool[] [TRUE, TRUE, TRUE, FALSE, TRUE] ("XMIT") bool[] [TRUE, TRUE, FALSE, FALSE, TRUE] ("XMIT") bool[] [TRUE, TRUE, FALSE, FALSE, TRUE] ("XMIT") bool[] [TRUE, TRUE, FALSE, FALSE, TRUE] ("XMIT") bool[] [TRUE, TRUE, FALSE, FALSE, TRUE] ("XMIT") bool[] [TRUE, TRUE, TRUE, TRUE, TRUE] ("XMIT")] -> w454
                tunnel: [w500 w515 w530 w545 w560 w575 w592 w607 w622 w637 w650] -> w456
                frame "20 MHz Full Globe" {
                  w499 = T2 {"Transducer"=99, "Geo Focus"=25.8, "a (radius)"=4.5, "# of rings"=5, "kerf space "=0.1, "Center Freq"=20.0}  # Trans Geometry (mm)
                  w501 = u16 100  # Amp (V)
                  w502 = u16 18  # Gain (dB)
                  w503 = u16 20  # Freq (MHz)
                  # "New probe full eye"
                  n184 = Bundle("Freq (MHz)"=w503, "Amp (V)"=w501, "Gain (dB)"=w502) -> (w500:T6)  [unwired: 1 in]
                }
                frame "20 MHz Anterior" {
                  w514 = T2 {"Transducer"=99, "Geo Focus"=25.8, "a (radius)"=4.5, "# of rings"=5, "kerf space "=0.1, "Center Freq"=20.0}  # Trans Geometry (mm)
                  w516 = u16 100  # Amp (V)
                  w517 = u16 18  # Gain (dB)
                  w518 = u16 20  # Freq (MHz)
                  # "New probe full eye"
                  n185 = Bundle("Freq (MHz)"=w518, "Amp (V)"=w516, "Gain (dB)"=w517) -> (w515:T6)  [unwired: 1 in]
                }
                frame "20 MHz Posterior" {
                  w529 = T2 {"Transducer"=99, "Geo Focus"=25.8, "a (radius)"=4.5, "# of rings"=5, "kerf space "=0.1, "Center Freq"=20.0}  # Trans Geometry (mm)
                  w531 = u16 100  # Amp (V)
                  w532 = u16 18  # Gain (dB)
                  w533 = u16 20  # Freq (MHz)
                  # "New probe full eye"
                  n186 = Bundle("Freq (MHz)"=w533, "Amp (V)"=w531, "Gain (dB)"=w532) -> (w530:T6)  [unwired: 1 in]
                }
                frame "New 20 MHz Full Globe" {
                  w544 = T2 {"Transducer"=99, "Geo Focus"=15.0, "a (radius)"=3.0, "# of rings"=5, "kerf space "=0.1, "Center Freq"=20.0}  # Trans Geometry (mm)
                  w546 = u16 100  # Amp (V)
                  w547 = u16 18  # Gain (dB)
                  w548 = u16 20  # Freq (MHz)
                  # "New probe full eye"
                  n187 = Bundle("Freq (MHz)"=w548, "Amp (V)"=w546, "Gain (dB)"=w547) -> (w545:T6)  [unwired: 1 in]
                }
                frame "New 20 MHz Anterior" {
                  w559 = T2 {"Transducer"=99, "Geo Focus"=15.0, "a (radius)"=3.0, "# of rings"=5, "kerf space "=0.1, "Center Freq"=20.0}  # Trans Geometry (mm)
                  w561 = u16 100  # Amp (V)
                  w562 = u16 18  # Gain (dB)
                  w563 = u16 20  # Freq (MHz)
                  # "New probe full eye"
                  n188 = Bundle("Freq (MHz)"=w563, "Amp (V)"=w561, "Gain (dB)"=w562) -> (w560:T6)  [unwired: 1 in]
                }
                frame "New 20 MHz Posterior" {
                  w574 = T2 {"Transducer"=99, "Geo Focus"=15.0, "a (radius)"=3.0, "# of rings"=5, "kerf space "=0.1, "Center Freq"=20.0}  # Trans Geometry (mm)
                  w576 = u16 100  # Amp (V)
                  w577 = u16 18  # Gain (dB)
                  w578 = u16 20  # Freq (MHz)
                  # "New probe full eye"
                  n189 = Bundle("Freq (MHz)"=w578, "Amp (V)"=w576, "Gain (dB)"=w577) -> (w575:T6)  [unwired: 1 in]
                }
                frame "F2 40 MHz", Default {
                  w591 = T2 {"Transducer"=0, "Geo Focus"=12.0, "a (radius)"=3.0, "# of rings"=5, "kerf space "=0.1, "Center Freq"=40.0}  # Trans Geometry (mm)
                  w593 = u16 0  # Amp (V)
                  w594 = u16 6  # Gain (dB)
                  w595 = u16 40  # Freq (MHz)
                  n190 = Bundle("Freq (MHz)"=w595, "Amp (V)"=w593, "Gain (dB)"=w594) -> (w592:T6)  [unwired: 1 in]
                }
                frame "F2 40 MHz Deep" {
                  w606 = T2 {"Transducer"=0, "Geo Focus"=12.0, "a (radius)"=3.0, "# of rings"=5, "kerf space "=0.1, "Center Freq"=40.0}  # Trans Geometry (mm)
                  w608 = u16 0  # Amp (V)
                  w609 = u16 6  # Gain (dB)
                  w610 = u16 40  # Freq (MHz)
                  n191 = Bundle("Freq (MHz)"=w610, "Amp (V)"=w608, "Gain (dB)"=w609) -> (w607:T6)  [unwired: 1 in]
                }
                frame "F3 20 MHz" {
                  w621 = T2 {"Transducer"=1, "Geo Focus"=31.0, "a (radius)"=5.0, "# of rings"=5, "kerf space "=0.1, "Center Freq"=20.0}  # Trans Geometry (mm)
                  w623 = u16 0  # Amp (V)
                  w624 = u16 6  # Gain (dB)
                  w625 = u16 20  # Freq (MHz)
                  n192 = Bundle("Freq (MHz)"=w625, "Amp (V)"=w623, "Gain (dB)"=w624) -> (w622:T6)  [unwired: 1 in]
                }
                frame "F3 20 MHz Deep" {
                  w636 = T2 {"Transducer"=1, "Geo Focus"=31.0, "a (radius)"=5.0, "# of rings"=5, "kerf space "=0.1, "Center Freq"=20.0}  # Trans Geometry (mm)
                  w638 = u16 0  # Amp (V)
                  w639 = u16 6  # Gain (dB)
                  w640 = u16 20  # Freq (MHz)
                  n193 = Bundle("Freq (MHz)"=w640, "Amp (V)"=w638, "Gain (dB)"=w639) -> (w637:T6)  [unwired: 1 in]
                }
                frame "Aviso Probe" {
                  w649 = T2 {"Transducer"=0, "Geo Focus"=12.0, "a (radius)"=3.0, "# of rings"=5, "kerf space "=0.1, "Center Freq"=40.0}  # Trans Geometry (mm)
                  w651 = u16 0  # Amp (V)
                  w652 = u16 6  # Gain (dB)
                  w653 = u16 40  # Freq (MHz)
                  # "Test Case"
                  n194 = Bundle("Freq (MHz)"=w653, "Amp (V)"=w651, "Gain (dB)"=w652) -> (w650:T6)  [unwired: 1 in]
                }
              }
              n195 = property on="Daxsonics Settings" class="Clust (strict)"("Value"=w456) -> ()  [unwired: 2 in, 2 out]
              n196 = Bundle("XMIT"=w454, "XMIT"=w453) -> (w452:cluster{"XMIT":bool[], "XMIT":bool[]})  [unwired: 1 in]
              n197 = local write "Xmt/Rcv"(w452) -> ()
              n198 = Bundle By Name(cluster=w450, "Xmt/Rcv"=w452, "Focal Zones"="Focal Zones", "Trans Geometry (mm)"=w451, "Synth Foc?"=TRUE, "GPU?"="GPU?") -> (w449:T1)
              n199 = call "Set_Daxsonics_3Pulsers.vi"("Daxsonics Settings"=w456) -> ()  [unwired: 9 in]
              n200 = Unbundle By Name(w464) -> ("Offset delay (us)"=w463:dbl)
              n201 = Add(x=w463, y=w466) -> (x+y=w472:dbl)
              n202 = expression code="x*1E-6"(w472) -> (w473:dbl)
              n203 = case shown="\"NI Digitizer\"" w476 {
                tunnel: w464 -> [_ w480 _]
                tunnel: w467 -> [_ w484 _]
                tunnel: w473 -> [_ w483 _]
                tunnel: w468 -> [_ w482 _]
                tunnel: w469 -> [_ w481 _]
                frame "Acqiris Digitizer", Default {
                }
                frame "NI Digitizer" {
                  n204 = Unbundle By Name(w480) -> ("Digitizer ID Cluster.NI Instr Handles"=w479:refnum<k15>[])
                  n205 = for {
                    tunnel: T25 {"Source"=1, "Coupling"=0, "Slope"=0, "Level (mV)"=2500.0} ("Trigger Settings") -> [w498]
                    tunnel: w482 -> [w495]
                    tunnel: w484 -> [w493]
                    tunnel: w481 -> [w492]
                    tunnel: w483 -> [w489]
                    tunnel: w479 -> [w488] mode=indexing
                    n206 = call "NIconTrig.vi"("Trigger"=w498, "InstrumentID"=w488) -> ("error out"=w496:errorcluster, "dup id"=w497:refnum<k15>)  [unwired: 1 in, 1 out]
                    n207 = call <instrlib>:"niScope Configure Horizontal Timing.vi"("instrument handle"=w497, "number of records"=w492, "min sample rate"=w495, "reference position"=0.0, "error in"=w496, "min record length"=w493) -> ("instrument handle out"=w491:refnum<k15>, "error out"=w490:errorcluster)  [unwired: 1 in, 7 out]
                    n208 = property class="niScope"(reference=w491, error in=w490, "Trigger Delay"=w489, "Active Channel"="0,1", "Channel Enabled"=TRUE ("Vertical:Channel Enabled")) -> ()  [unwired: 2 out]
                  }
                }
                frame "LeCroy" {
                  # "Alazat Settings handled downstream"
                }
              }
              n209 = expression code="x*1E-6"(w468) -> (w471:dbl)
              n210 = Bundle By Name(cluster=w464, "Xtra Ann Trig delay (us)"="Xtra delay (us)", "lines per plane"=w469, "Samp Rate (Hz)"=w468, "rf points per line"=w467, "Digitizer delay (us)"=w466) -> (w465:T14)
              n211 = Decrement(x=w469) -> (x-1=w474:i32)
              n212 = Bundle(w471, w466, w467) -> (w470:cluster{dbl, dbl, i32})  [unwired: 1 in]
              n213 = Multiply(x=w474, y=w457) -> (x*y=w458:sgl)
              n214 = Bundle By Name(cluster=w462, "Total steps in line"=w458, "Distance between\nscan lines (um)"=w457, "overshoot cts"=w461, "RT fps"=w460) -> (w459:T31)
              n215 = flat-sequence {
                tunnel: w470 -> [w477]
                frame #0 {
                  n216 = property on="RF data Sampling" class="Clust (strict)"("Val(Sgnl)"=w477) -> ()  [unwired: 2 in, 2 out]
                }
                frame #1 {
                  n217 = property on="Image Scaling" class="RadioBtnsControl (strict)"("Val(Sgnl)"=T5."1:1\nAspect" ("Value (Signaling)")) -> ()  [unwired: 2 in, 2 out]
                }
              }
            }
            event "RF data Sampling", "c (m/s)": Value Change {
              n218 = event-data() -> ()  [unwired: 1 in, 3 out]
              n219 = Unbundle By Name(w665) -> ("StopN"=w689:refnum<notifier>)
              n220 = Unbundle("RF data Sampling") -> ("Sampling Rate"=w690:dbl, "Ref Delay (ms)"=w684:dbl, "rf points per line"=w685:i32)
              n221 = expression code="x*1E6"(w690) -> (w683:dbl)
              n222 = Bundle By Name(cluster=w686, "Samp Rate (Hz)"=w683, "Digitizer delay (us)"=w684, "rf points per line"=w685) -> (w667:T14)
              n223 = case shown="True" w688 {
                tunnel: w689 -> [_ w700]
                frame False {
                }
                frame True {
                  n224 = flat-sequence {
                    tunnel: w700 -> [w701]
                    frame #0 {
                      n225 = Send Notification(notification=TRUE, notifier=w701) -> ()  [unwired: 1 in, 2 out]
                    }
                    frame #1 {
                      n226 = Wait (ms)(milliseconds to wait=u32 500) -> ()  [unwired: 1 out]
                    }
                  }
                }
              }
              n227 = Unbundle By Name(w666) -> ("Distance between\nscan lines (um)"=w671:sgl)
              n228 = expression code="x/1000"("c (m/s)") -> (w668:dbl)
              n229 = Unbundle By Name(w667) -> ("lines per plane"=w682:i32)
              n230 = flat-sequence {
                tunnel: w681 -> [w693]
                tunnel: w667 -> [w694]
                tunnel: [w694] -> w674
                tunnel: [w693] -> w673
                tunnel: w668 -> [w692]
                tunnel: [w692] -> w669
                tunnel: [w697] -> w680
                tunnel: w674 -> [w699]
                tunnel: w673 -> [w698]
                tunnel: w669 -> [w696]
                tunnel: w666 -> [w695]
                frame #0 {
                }
                frame #1 {
                  n231 = call "PlotScalingParams.vi"("Motion Settings In"=w695, "c mm/mics"=w696, "Digitizer Settings"=w699, "Scan Axis"=w698) -> ("Cluster"=w697:T40)  [unwired: 5 in, 2 out]
                }
              }
              n232 = global write "MotionGlobals.vi" "c mm/mics"(w668) -> ()
              n233 = Decrement(x=w682) -> (x-1=w691:i32)
              n234 = Multiply(x=w691, y=w671) -> (x*y=w672:sgl)
              n235 = Bundle By Name(cluster=w666, "Total steps in line"=w672) -> (w670:T31)
              n236 = Unbundle By Name(w680) -> ("X Scale Offset"=w679:dbl, "X Scale Multi"=w677:dbl, "Y Scale Offset"=w676:dbl, "Y Scale Multi"=w675:dbl)
              n237 = property on="Raw data" class="IntGraph (strict)"("X Scale.Offset and Multiplier:Offset"=w679, "X Scale.Offset and Multiplier:Multiplier"=w677, "Y Scale.Offset and Multiplier:Offset"=w676, "Y Scale.Offset and Multiplier:Multiplier"=w675) -> ()  [unwired: 2 in, 2 out]
            }
            event "Dig Scale": Value Change {
              n238 = event-data() -> ("NewVal"=w710:dbl)  [unwired: 1 in]
              n239 = Unbundle By Name(w713) -> ("StopN"=w712:refnum<notifier>)
              n240 = case shown="True" w709 {
                tunnel: w712 -> [_ w741]
                tunnel: [_ w740] -> w711
                frame False {
                }
                frame True {
                  n241 = flat-sequence {
                    tunnel: w741 -> [w743]
                    tunnel: [w742] -> w739
                    tunnel: [w745] -> w740
                    tunnel: w739 -> [w745]
                    frame #0 {
                      n242 = Send Notification(notification=TRUE, notifier=w743) -> (error out=w742:errorcluster)  [unwired: 1 in, 1 out]
                    }
                    frame #1 {
                      n243 = Wait (ms)(milliseconds to wait=u32 1000) -> ()  [unwired: 1 out]
                    }
                  }
                }
              }
              n244 = case shown="\"AlazarTech\"" w708 {
                tunnel: w706 -> [w714 w715 w726]
                tunnel: w711 -> [_ w718 _]
                tunnel: w710 -> [_ w717 w728]
                tunnel: [w714 w715 w727] -> w707
                frame "Acqiris Digitizer", Default {
                }
                frame "NI Digitizer" {
                  n245 = Unbundle By Name(w715) -> ("Digitizer ID Cluster.NI Instr Handles"=w716:refnum<k15>[])
                  n246 = for {
                    tunnel: w717 -> [w721]
                    tunnel: w718 -> [w720]
                    tunnel: w716 -> [w719] mode=indexing
                    n247 = property class="niScope"(reference=w719, error in=w720, "Active Channel"="0,1", "Vertical Range"=w721) -> ()  [unwired: 2 out]
                  }
                }
                frame "AlazarTech" {
                  n248 = Unbundle By Name(w726) -> ("Digitizer ID Cluster.Acqiris/Alazar/SP ID"=w723:u32[])
                  n249 = Bundle By Name(cluster=w726, "Voltage Scale"=w728) -> (w727:T14)
                  n250 = Array Size(array=w723) -> (size(s)=w724:i32)
                  n251 = case shown="2" w724 {
                    tunnel: [w737 w738] -> w725
                    frame 2 {
                      w737 = u8[] [1, 2] items=["A"=1, "B"=2, "C"=4, "D"=8]
                    }
                    frame 1, Default {
                      w738 = u8[] [1, 2, 4, 8] items=["A"=1, "B"=2, "C"=4, "D"=8]
                    }
                  }
                  n252 = Bundle By Name(cluster=T26 {"Voltage Scale"=0.0, "Offset"=0.0, "Coupling"=2} ("V scale"), "Voltage Scale"=w728) -> (w730:T26)
                  n253 = for {
                    tunnel: w730 -> [w733]
                    tunnel: w725 -> [w732]
                    tunnel: w723 -> [w731] mode=indexing
                    n254 = for {
                      tunnel: w731 -> [w736]
                      tunnel: w733 -> [w735]
                      tunnel: w732 -> [w734] mode=indexing
                      n255 = call "Alazar_ChannelConfig - ATS-SDK.vi"("V scale"=w735, "Channel"=w734, "Handle in"=w736) -> ()  [unwired: 2 in, 3 out]
                    }
                  }
                }
              }
            }
            event "Daxsonics Settings": Value Change {
              n256 = event-data() -> ("NewVal"=w748:T6)  [unwired: 1 in]
              n257 = call "Set_Daxsonics_3Pulsers.vi"("Daxsonics Settings"=w748) -> ()  [unwired: 9 in]
            }
            event "Xmt/Rcv": Value Change {
              n258 = event-data() -> ("NewVal"=w752:cluster{"XMIT":bool[], "RCV":bool[]}, "OldVal.RCV"=w758:bool[])  [unwired: 1 in]
              n259 = Boolean Array To Number(Boolean array=w758) -> (number=w759:u32)
              n260 = case shown="1, Default" w759 {
                tunnel: w760 -> [_ w764]
                tunnel: w757 -> [_ w762]
                tunnel: [_ w762] -> w756
                frame 0 {
                  n261 = One Button Dialog(message="Must have at least one element active on transmit and receive.") -> ()  [unwired: 1 in, 1 out]
                }
                frame 1, Default {
                  n262 = Unbundle By Name(w764) -> ("StopN"=w763:refnum<notifier>)
                  n263 = case shown="True" w762 {
                    tunnel: w763 -> [_ w765]
                    frame False {
                    }
                    frame True {
                      n264 = flat-sequence {
                        tunnel: w765 -> [w766]
                        frame #0 {
                          n265 = Send Notification(notification=TRUE, notifier=w766) -> ()  [unwired: 1 in, 2 out]
                        }
                        frame #1 {
                          n266 = Wait (ms)(milliseconds to wait=u32 1000) -> ()  [unwired: 1 out]
                        }
                      }
                    }
                  }
                }
              }
              n267 = Bundle By Name(cluster=w753, "Xmt/Rcv"=w752) -> (w751:T1)
            }
            event "ExitSendCmd": Value Change {
              n268 = event-data() -> ()  [unwired: 1 in, 5 out]
              n269 = Unbundle By Name(w773) -> ("StopN"=w772:refnum<notifier>)
              n270 = flat-sequence {
                tunnel: w772 -> [w775]
                frame #0 {
                  n271 = Send Notification(notification=TRUE, notifier=w775) -> ()  [unwired: 1 in, 2 out]
                }
                frame #1 {
                  n272 = Wait (ms)(milliseconds to wait=u32 100) -> ()  [unwired: 1 out]
                }
              }
            }
            event "File Name": Value Change {
              n273 = event-data() -> ("NewVal"=w782:string)  [unwired: 1 in]
              n274 = case shown="True" TRUE {
                tunnel: w782 -> [_ w785]
                frame False {
                }
                frame True {
                  # "Pull all named files"
                  n275 = Concatenate Strings(w785, "*") -> (w788:string)
                  n276 = global read "MotionGlobals.vi" "SavePath"() -> (w783:path)
                  n277 = List Folder(path=w783, pattern=w788) -> (filenames=w787:string[])  [unwired: 1 in, 4 out]
                  n278 = Array Size(array=w787) -> (size(s)=w784:i32)
                  n279 = case shown="1, Default" w784 {
                    frame 0 {
                    }
                    frame 1, Default {
                      n280 = One Button Dialog(message="File name has been used already. Select a new file name.") -> ()  [unwired: 1 in, 1 out]
                    }
                  }
                }
              }
            }
            event "Patient Info": Value Change {
              n281 = event-data() -> ()  [unwired: 1 in, 1 out]
              n282 = call "Info.vi"("Patient Info In"=w795) -> ("NewCase?"=w793:bool, "FileName"=→"File Name":string, "Patient Info Out"=w798:T41)  [unwired: 8 in]
              n283 = local write "Patient Info"(FALSE ("Patient Info")) -> ()
              n284 = Unbundle By Name(w798) -> ("Plane"=w797:i8)
              n285 = local write "Plane"(w797) -> ()
              n286 = case shown="True" w793 {
                frame False {
                }
                frame True {
                  # "Rest Letter Index"
                  n287 = local write "append letter"(i8 65 ("append letter")) -> ()
                }
              }
            }
            event "Plane": Mouse Up; "Scan Location": Value Change {
              n288 = event-data() -> ()  [unwired: 1 in, 4 out]
              n289 = global read "PatientGlobals.vi" "Patient Info"() -> (w802:T41)
              n290 = Bundle By Name(cluster=w802, "Plane"="Plane", "Scan Location"="Scan Location") -> (w801:T41)
              n291 = global write "PatientGlobals.vi" "Patient Info"(w801) -> ()
            }
            event "View Queue": Value Change {
              # "Save files baed on queue selection"
              n292 = event-data() -> ()  [unwired: 1 in, 1 out]
              n293 = Unbundle By Name(w814) -> ("LastNBMPQ"=w815:refnum<queue>)
              n294 = call "ViewQueue.vi"("Image queue"=w815) -> ("Slider Indexes"=w811:cluster{i16, i16, i16}, "Save?"=w812:bool)  [unwired: 3 in]
              n295 = case shown="True" w812 {
                tunnel: w814 -> [_ w822]
                tunnel: w813 -> [_ w821]
                tunnel: w811 -> [_ w820]
                tunnel: w810 -> [_ w819]
                tunnel: w807 -> [_ w816]
                frame False {
                }
                frame True {
                  n296 = call "SaveQueueN.vi"("Ann Array Params"=w816, "File Name"=w819, "bits A/D"=u16 11, "append letter"=w821, "Qs and Notis"=w822, "Slider Indexes"=w820) -> ("append letter out"=w818:i8)  [unwired: 5 in]
                  n297 = local write "append letter"(w818) -> ()
                }
              }
            }
            event "Save All Queue": Value Change {
              w828 = i16 1
              # "Save 1 to N"
              n298 = event-data() -> ()  [unwired: 1 in, 5 out]
              n299 = Bundle(w828, w828, "N"="N") -> (w827:cluster{i16, i16, "N":u8})  [unwired: 1 in]
              n300 = local write "Save All Queue"(FALSE ("Save Last N")) -> ()
              n301 = call "SaveQueueN.vi"("Ann Array Params"=w823, "File Name"=w834, "bits A/D"=u16 11, "append letter"=w831, "Qs and Notis"=w832, "Slider Indexes"=w827) -> ("append letter out"=w830:i8)  [unwired: 5 in]
              n302 = local write "append letter"(w830) -> ()
            }
            event "Save All Real Time": Value Change {
              n303 = event-data() -> ("NewVal"=w838:bool)  [unwired: 1 in]
              n304 = case shown="False" w838 {
                tunnel: w839 -> [w840 _]
                frame False {
                  n305 = Increment(x=w840) -> (x+1=w841:i8)
                  n306 = local write "append letter"(w841) -> ()
                }
                frame True {
                }
              }
            }
            event "Save Raw": Value Change {
              n307 = event-data() -> ()  [unwired: 1 in, 1 out]
              n308 = Unbundle By Name(w850) -> ("SaveRawN"=w849:refnum<notifier>)
              n309 = global read "MotionGlobals.vi" "SavePath"() -> (w848:path)
              n310 = Build Path(base path=w848, name or relative path="Raw") -> (appended path=w845:path)
              n311 = File/Directory Info(path=w845) -> (error out=w846:errorcluster)  [unwired: 1 in, 6 out]
              n312 = Send Notification(notification="Save Raw", notifier=w849) -> ()  [unwired: 1 in, 2 out]
              n313 = case shown="Error" w846 {
                tunnel: w845 -> [_ w852]
                frame No Error {
                }
                frame Error {
                  n314 = Create Folder(path (use dialog)=w852) -> ()  [unwired: 2 in, 3 out]
                }
              }
            }
            event "Center": Value Change {
              n315 = event-data() -> ()  [unwired: 1 in, 5 out]
              n316 = property on="Raw data" class="IntGraph (strict)"() -> ("XScale.Maximum"=w866:dbl, "XScale.Minimum"=w865:dbl, "YScale.Maximum"=w864:dbl, "YScale.Minimum"=w863:dbl)  [unwired: 2 in, 2 out]
              n317 = Add(x=w866, y=w865) -> (x+y=w862:dbl)
              n318 = Add(x=w864, y=w863) -> (x+y=w861:dbl)
              n319 = expression code="x/2"(w862) -> (w860:dbl)
              n320 = expression code="x/2"(w861) -> (w859:dbl)
              n321 = Bundle(w860, w859) -> (w856:cluster{dbl, dbl})  [unwired: 1 in]
              n322 = property on="Raw data" class="IntGraph (strict)"("Active Cursor"=u32 0, "Cursor.Cursor Position"=w856, "Active Cursor"=u32 1, "Cursor.Cursor Position"=w856) -> ()  [unwired: 2 in, 2 out]
            }
            event "Visible": Value Change {
              n323 = event-data() -> ("NewVal"=w870:bool)  [unwired: 1 in, 4 out]
              n324 = property on="Raw data" class="IntGraph (strict)"("Active Cursor"=u32 0, "Cursor.Visible"=w870, "Active Cursor"=u32 1, "Cursor.Visible"=w870) -> ()  [unwired: 2 in, 2 out]
            }
            event "Raw data": Cursor Move {
              n325 = event-data() -> ()  [unwired: 1 in, 2 out]
              n326 = property on="Raw data" class="IntGraph (strict)"("Active Cursor"=u32 0, "Active Cursor"=u32 1) -> ("Cursor.Cursor Position"=w881:T42, "Cursor.Cursor Position"=w886:T42)  [unwired: 2 in, 2 out]
              n327 = Subtract(x=w881, y=w886) -> (x-y=w885:T42)
              n328 = Unbundle(w885) -> ("Cursor X"=w884:dbl, "Cursor Y"=w876:dbl)
              n329 = Re/Im To Polar(2:w876, 3:w884) -> (1:w877:dbl)  [unwired: 1 out]
              n330 = Number To Fractional String(number=w877, precision (6)=i16 2) -> (F-format string=w880:string)  [unwired: 2 in]
              n331 = Concatenate Strings(w880, " mm") -> (w878:string)
              n332 = property on="Raw data" class="IntGraph (strict)"("Active Cursor"=u32 0, "Cursor.Cursor Name"=w878) -> ()  [unwired: 2 in, 2 out]
            }
            event "Image Scaling": Value Change {
              n333 = event-data() -> ("NewVal"=w892:T5)  [unwired: 1 in]
              n334 = case shown="\"1:1\\nAspect\", Default" w892 {
                tunnel: w894 -> [w900 _ _]
                tunnel: w893 -> [w899 w927 _]
                tunnel: w891 -> [w897 _ _]
                frame "1:1\nAspect", Default {
                  w898 = u8 1 ("X Scale.Scale Fit")
                  n335 = property on="Raw data" class="IntGraph (strict)"("XScale.ScaleFit"=w898, "YScale.ScaleFit"=w898) -> ("X Scale.Offset and Multiplier:Multiplier"=w912:dbl, "Y Scale.Offset and Multiplier:Multiplier"=w911:dbl)  [unwired: 2 in, 2 out]
                  n336 = Unbundle By Name(w897) -> ("lines per plane"=w896:i32, "rf points per line"=w895:i32)
                  n337 = Multiply(x=w896, y=w912) -> (x*y=w910:dbl)
                  n338 = Multiply(x=w911, y=w895) -> (x*y=w909:dbl)
                  n339 = Unbundle(w900) -> ("Width"=w904:u32, "Height"=w902:u32)
                  n340 = Divide(x=w904, y=w910) -> (x/y=w908:dbl)
                  n341 = Divide(x=w902, y=w909) -> (x/y=w907:dbl)
                  n342 = Divide(x=w908, y=w907) -> (x/y=w903:dbl)
                  n343 = Greater?(x=w903, y=1.0) -> (0:w906:bool)
                  n344 = case shown="True" w906 {
                    tunnel: w904 -> [_ w926]
                    tunnel: w903 -> [w919 w925]
                    tunnel: w902 -> [w918 _]
                    tunnel: w899 -> [w913 w924]
                    tunnel: [w914 w920] -> w901
                    frame False {
                      n345 = Unbundle By Name(w913) -> ("Top"=w917:i16)
                      n346 = Multiply(x=w918, y=w919) -> (x*y=w915:dbl)
                      n347 = Add(x=w917, y=w915) -> (x+y=w916:dbl)
                      n348 = Bundle By Name(cluster=w913, "Bottom"=w916) -> (w914:T10)
                    }
                    frame True {
                      n349 = Unbundle By Name(w924) -> ("Left"=w922:i16)
                      n350 = Divide(x=w926, y=w925) -> (x/y=w923:dbl)
                      n351 = Add(x=w922, y=w923) -> (x+y=w921:dbl)
                      n352 = Bundle By Name(cluster=w924, "Right"=w921) -> (w920:T10)
                    }
                  }
                  n353 = property on="Raw data" class="IntGraph (strict)"("Plot Bounds"=w901) -> ()  [unwired: 2 in, 2 out]
                }
                frame "Fill\nSpace" {
                  (unwired) T10 {"Left"=666, "Top"=-99, "Right"=1566, "Bottom"=695} ("Plot Area Bounds")
                  n354 = property on="Raw data" class="IntGraph (strict)"("Plot Bounds"=w927) -> ()  [unwired: 2 in, 2 out]
                }
                frame "Auto\nScale" {
                  w928 = u8 1 ("X Scale.Scale Fit")
                  n355 = property on="Raw data" class="IntGraph (strict)"("XScale.ScaleFit"=w928, "YScale.ScaleFit"=w928) -> ()  [unwired: 2 in, 2 out]
                }
              }
            }
            event "Scale (dB)": Value Change {
              n356 = event-data() -> ("NewVal"=w936:cluster{i32, i32})  [unwired: 1 in, 4 out]
              n357 = Unbundle(w936) -> (w934:i32, w933:i32)
              n358 = property on="Raw data" class="IntGraph (strict)"() -> ("ZScale.Range"=w935:T43)  [unwired: 2 in, 2 out]
              n359 = Bundle By Name(cluster=w935, "Minimum"=w933, "Maximum"=w934) -> (w932:T43)
              n360 = property on="Raw data" class="IntGraph (strict)"("ZScale.Range"=w932) -> ()  [unwired: 2 in, 2 out]
            }
            event "Adjust fps (%)": Value Change {
              n361 = event-data() -> ()  [unwired: 1 in, 2 out]
              n362 = case shown="\"NI 735x\"" w940 {
                tunnel: w942 -> [w944 _]
                tunnel: w941 -> [w943 _]
                frame "NI 735x" {
                  n363 = disable-structure shown="Disabled" {
                    disable-tunnel: "Adjust fps (%)" -> [w948 _]
                    disable-tunnel: w944 -> [w947 _]
                    disable-tunnel: w943 -> [w946 _]
                    frame Disabled {
                      n364 = call <vilib>:"Load Velocity Override.flx"("Override  Percentage (100%)"=w948, "Axis or Vector Space"=w946, "Board ID"=w947) -> ()  [unwired: 4 in, 3 out]
                    }
                    frame Enabled {
                    }
                  }
                }
                frame "No Motion Card", Default {
                }
              }
            }
            event "Accel": Value Change {
              n365 = event-data() -> ("NewVal"=w953:dbl)  [unwired: 1 in]
              n366 = case shown="\"NI 735x\", Default" w952 {
                tunnel: w955 -> [w958 _]
                tunnel: w954 -> [w957 _]
                tunnel: w953 -> [w956 _]
                frame "NI 735x", Default {
                  n367 = disable-structure shown="Disabled" {
                    disable-tunnel: w958 -> [w961 _]
                    disable-tunnel: w957 -> [w960 _]
                    disable-tunnel: w956 -> [w959 _]
                    frame Disabled {
                      n368 = call "Load Acceleration/Deceleration.flx"("Acceleration (100000)"=w959, "Axis or Vector Space"=w960, "Board ID"=w961) -> ()  [unwired: 4 in, 3 out]
                    }
                    frame Enabled {
                    }
                  }
                }
                frame "No Motion Card" {
                }
              }
            }
            event "Gate Length", "LowTime": Value Change {
              n369 = event-data() -> ()  [unwired: 1 in, 1 out]
              n370 = call "FrameSync.vi"("LowTime"="LowTime", "Gate Length"="Gate Length", "Main Digitizer"=w965) -> ()  [unwired: 7 in, 2 out]
            }
            event "Flush Queue": Value Change {
              n371 = event-data() -> ()  [unwired: 1 in, 6 out]
              n372 = Unbundle By Name(w973) -> ("LastNQ"=w972:refnum<queue>, "LastNBMPQ"=w971:refnum<queue>)
              n373 = Flush Queue(queue=w972) -> ()  [unwired: 1 in, 3 out]
              n374 = Flush Queue(queue=w971) -> ()  [unwired: 1 in, 3 out]
            }
          }
          n375 = Or(x=w338, y=w336) -> (x .or. y?=w337:bool)
        }
      }
      n376 = global write "DigitizerGlobals.vi" "Digitizer Settings"(w219) -> ()
      n377 = global write "MotionGlobals.vi" "Motion Settings"(w220) -> ()
      "append letter" <- i8 65
    }
    frame #6 {
      w979 = TRUE ("force destroy? (F)")
      n378 = Unbundle By Name(w977) -> ("DataBufferQ"=w983:refnum<queue>, "LastNQ"=w982:refnum<queue>, "LastNBMPQ"=w981:refnum<queue>, "SaveRawN"=w978:refnum<notifier>, "StopN"=w980:refnum<notifier>)
      n379 = case shown="True" FALSE {
        tunnel: w986 -> [_ w988]
        tunnel: w985 -> [_ w987]
        frame False {
        }
        frame True {
          n380 = property on="Raw data" class="IntGraph (strict)"("Plot Bounds"=w988, "Plot Area Size"=w987) -> ()  [unwired: 2 in, 2 out]
        }
      }
      n381 = Release Queue(queue=w983, force destroy? (F)=w979) -> ()  [unwired: 1 in, 3 out]
      n382 = Release Queue(queue=w982, force destroy? (F)=w979) -> ()  [unwired: 1 in, 3 out]
      n383 = Release Notifier(notifier=w980, force destroy? (F)=w979) -> ()  [unwired: 1 in, 3 out]
      n384 = Release Queue(queue=w981, force destroy? (F)=w979) -> ()  [unwired: 1 in, 3 out]
      n385 = Release Notifier(notifier=w978, force destroy? (F)=w979) -> ()  [unwired: 1 in, 3 out]
      n386 = case shown="\"NI Digitizer\"" w976 {
        tunnel: w974 -> [_ w990]
        frame "Acqiris Digitizer", Default {
        }
        frame "NI Digitizer" {
          n387 = Unbundle By Name(w990) -> ("Digitizer ID Cluster.NI Instr Handles"=w989:refnum<k15>[])
          n388 = for {
            tunnel: w989 -> [w991] mode=indexing
            n389 = call <instrlib>:"niScope Close.vi"("instrument handle"=w991) -> ()  [unwired: 1 in, 14 out]
          }
        }
      }
      n390 = local write "Save All Real Time"(FALSE ("Save CineLoop")) -> ()
    }
  }
